vi "SR Speckle.vi"() -> ()   [LabVIEW 2012]
uses:
  user.lib/SpectralRadar.llb/Coloring.lvclass
  user.lib/SpectralRadar.llb/Colored Data.lvclass
  user.lib/SpectralRadar.llb/Colorscheme Selection.ctl
  user.lib/SpectralRadar.llb/Data.lvclass
  user.lib/SpectralRadar.llb/Specle Variance Type.ctl
  <vilib>/Utility/error.llb/DialogType.ctl
  user.lib/SpectralRadar.llb/Coloring Byteorder.ctl
  user.lib/SpectralRadar.llb/Probe Parameter Int Selection.ctl
  user.lib/SpectralRadar.llb/Processing Parameter Int Selection.ctl
  user.lib/SpectralRadar.llb/Data Export Format Selection.ctl
  user.lib/SpectralRadar.llb/Colored Data Export Format Selection.ctl
  user.lib/SpectralRadar.llb/Normal Direction Selection.ctl
  user.lib/SpectralRadar.llb/Calibration Selection.ctl
  user.lib/SpectralRadar.llb/Data Analyzation Selection.ctl
  user.lib/SpectralRadar.llb/set Complex Scan Output.vi
  user.lib/SpectralRadar.llb/set Scan Output.vi
  user.lib/SpectralRadar.llb/display Data 2D.vi
  user.lib/SpectralRadar.llb/OCT Device.lvclass
  user.lib/SpectralRadar.llb/LabVIEW Helper.lvlib
  user.lib/SpectralRadar.llb/Processing.lvclass
  user.lib/SpectralRadar.llb/Probe.lvclass
  user.lib/SpectralRadar.llb/Scan Pattern.lvclass
  user.lib/SpectralRadar.llb/Settings.lvclass
  user.lib/SpectralRadar.llb/Raw Data.lvclass
  user.lib/SpectralRadar.llb/FileSelection.lvlib
  user.lib/SpectralRadar.llb/Complex Data.lvclass
  user.lib/SpectralRadar.llb/Speckle Variance.lvclass
  user.lib/SpectralRadar.llb/Post Processing.lvlib
  user.lib/SpectralRadar.llb/FullRange.lvclass
panel:
  in  "Filter 3":bool
  in  "Filter 2":bool
  in  "Filter":bool
  in  "Filter Options":bool
  in  "Variance Type":T1
  in  "Averaging Axially":i32=1 min=1 max=10 step=1
  in  "Averaging Fast Axis":i32=1 min=1 max=10 step=1
  in  "Averaging Slow Axis":i32=3 min=1 max=10 step=1
  out "Volume Variance":refnum<class "Data.lvclass">
  out "Volume Mean":refnum<class "Data.lvclass">
  in  "Opacity":sgl(slide) scale=0.0..1.0
  in  "Shift Y [mm]":dbl
  in  "Shift X [mm]":dbl
  in  "Color Scheme":T2
  in  "Options":bool
  out "Colored Data":refnum<class "Colored Data.lvclass">
  out "Coloring":refnum<class "Coloring.lvclass">
  in  "Angle [rad]":dbl
  in  "Averaging-Binning-Ratio":dbl(slide) caption="Averaging vs. Binning" min=0.0 max=1.0 step=1.0
  in  "Averaging*Binning":i32(slide)=1 caption="Quality" min=1 max=200 step=1 scale=1.0..200.0
  out "AutoSafe":bool
  out "Progress":i32(slide) max=20 scale=0.0..384.0
  in  "Tab Control":enum32{"B-Scan"}(tab)
  out "Variance Frame":sgl[][](graph)
  in  "Variance Boundaries":cluster{sgl, sgl}(slide)={72.22738, 40.64965} scale=0.0..144.0705108642578
  in  "Boundries":cluster{sgl, sgl}(slide)={72.22738, 40.64965} scale=-20.0..150.0
  out "Mean Frame":sgl[][](graph)
  in  "X":dbl(slide) max=2.0 scale=0.0..2.0
  in  "Y":dbl(slide) max=3.0 scale=0.0..2.0
  in  "Z":dbl(slide) max=1.600000023841858 scale=0.0..5.12 scale format="%#_2g"
  in  "Export Format":T3(ring)
  out "Image":T4(plugin-control)
  out "Reference Intensity":sgl(slide) min=0 max=1 scale=0.0..1.0
  in  "Brightness":sgl(slide)=0.49673203 caption="Sharpness" min=0 max=1 scale=0.0..1.0
  in  "Contrast":sgl(slide)=0.53594774 caption="Sharpness" min=0 max=1 scale=0.0..1.0
  in  "Saturation":sgl(slide)=0.5294118 caption="Sharpness" min=0 max=1 scale=0.0..1.0
  in  "Light":i32(slide) min=0 max=100 step=1 scale=0.0..100.0
  in  "Description":string
  in  "Test Mode":bool
  out "Test Mode Indicator":bool
  in  "Window":T5(ring)
  out "FrameRate":sgl format="%#_3g"
  out "SpacingZ":dbl
  in  "Range Y [mm]":dbl=3.5999999046325684 caption="Bereich [mm]" min=0.0 max=10.0 step=0.05000000074505806 format="%_3f"
  out "Spacing Y [µm]":dbl=40.0 min=1.0 max=500.0 step=1.0 format="%#_3g"
  in  "Number Scans Y":i32=50 min=10 max=1000 step=1
  in  "Save":bool
  in  "Recalibrate":bool
  in  "Range X [mm]":dbl=2.5999999046325684 caption="Bereich [mm]" min=0.05000000074505806 max=10.0 step=0.05000000074505806 format="%_3f"
  out "Spacing X [µm]":dbl=2.0 min=1.0 max=500.0 step=1.0 format="%#_3g"
  in  "Number Scans X":i32=500 min=100 max=2000 step=1
  in  "Measure":bool
  in  "QuitApp":bool
  # "Stability"
  # "SNR"
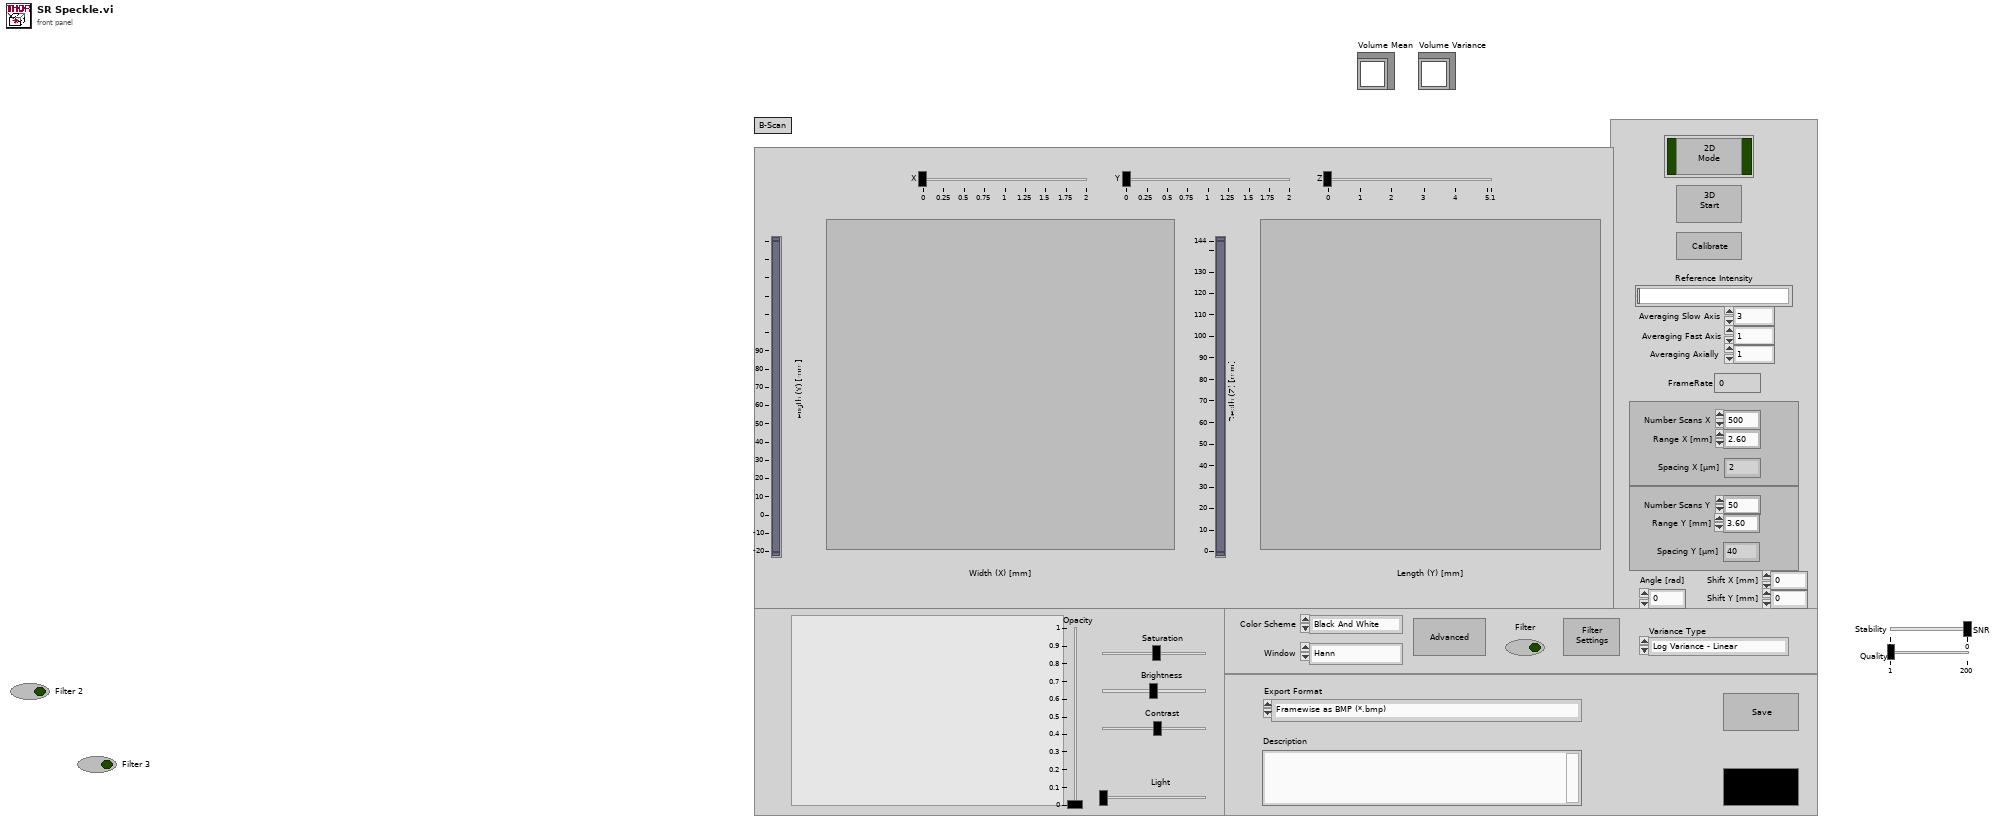
[diagram p1: front panel]
types:
  T1 = typedef "Speckle Variance.lvclass/Specle Variance Type.ctl" = enum16{"Log Variance - Linear", "Log Variance - Log", "Linear Variance - Linear", "Linear Variance - Log", "Complex Variance - Linear", "Complex Variance - Log"}
  T2 = typedef "Coloring.lvclass/Colorscheme Selection.ctl" = enum16{"Black And White", "Inverted Black And White", "Color", "Black and Orange", "Black and Red", "Doppler Phase Coloring"}
  T3 = enum16{"Framewise as BMP (*.bmp)", "Framewise as JPG (*.jpg)", "Framewise as PNG (*.png)", "Raw binary floating point (*.raw)", "VFF (*.vff)", "VTK (*.vtk)", "Flexible Image Transport System (*.fits)"}
  T4 = typedef "IMAQ Image.ctl" = refnum<image>
  T5 = enum16{"Hann", "Hamming", "Gauss", "Tapered Cosine", "Blackman", "4 Term B-Harris"}
  T6 = typedef "Coloring.lvclass/Coloring Byteorder.ctl" = enum16{"RGBA32", "BGRA32", "ARGB32", ""}
  T7 = enum16{"Full Well Capacity", "z Spacing", "z Range", "Dynamc Range Min [dB]", "Dynamic Range Low [dB]", "Dynamic Range High [dB]", "Dynamic Range Max [dB]"}
  T8 = typedef "Processing.lvclass/Processing Parameter Int Selection.ctl" = enum32{"Spectrum Averaging", "A-Scan Averaging", "B-Scan Averaging", "Zero Padding", "Number of Threads", "Fourier Averaging"}
  T9 = typedef "Probe.lvclass/Probe Parameter Int Selection.ctl" = enum16{"Apodization Cycles", "Oversampling", "Oversampling Slow Axis", "Speckle Reduction"}
  T10 = typedef "Data.lvclass/Data Export Format Selection.ctl" = enum16{"SRM (Spectral Radar Metafile)", "RAW", "CSV", "TXT", "Table TXT", "Fits", "VFF", "VTK", "TIFF"}
  T11 = typedef "Colored Data.lvclass/Colored Data Export Format Selection.ctl" = enum16{"SRM (Spectral Radar Metafile)", "RAW", "BMP", "PNG", "JPG", "PDF", "TIFF"}
  T12 = enum16{"Asynchronous Continuous", "Asynchronous Finite", "Synchronous"}
  T13 = typedef "Data.lvclass/Normal Direction Selection.ctl" = enum16{"Direction 1", "Direction 2", "Direction 3"}
  T14 = enum8{"Enabled", "Disabled", "Disabled and Grayed Out"}
  T15 = typedef "Processing.lvclass/Calibration Selection.ctl" = enum16{"Offset Errors", "Apodization Spectrum", "Apodization Vector", "Dispersion", "Chirp", "Extended Adjust", "Fixed Pattern"}
  T16 = typedef "Data.lvclass/Data Analyzation Selection.ctl" = enum16{"Min", "Mean", "Max"}
  T17 = typedef "DialogType.ctl" = u16
  T18 = typedef "Image Type" = u32
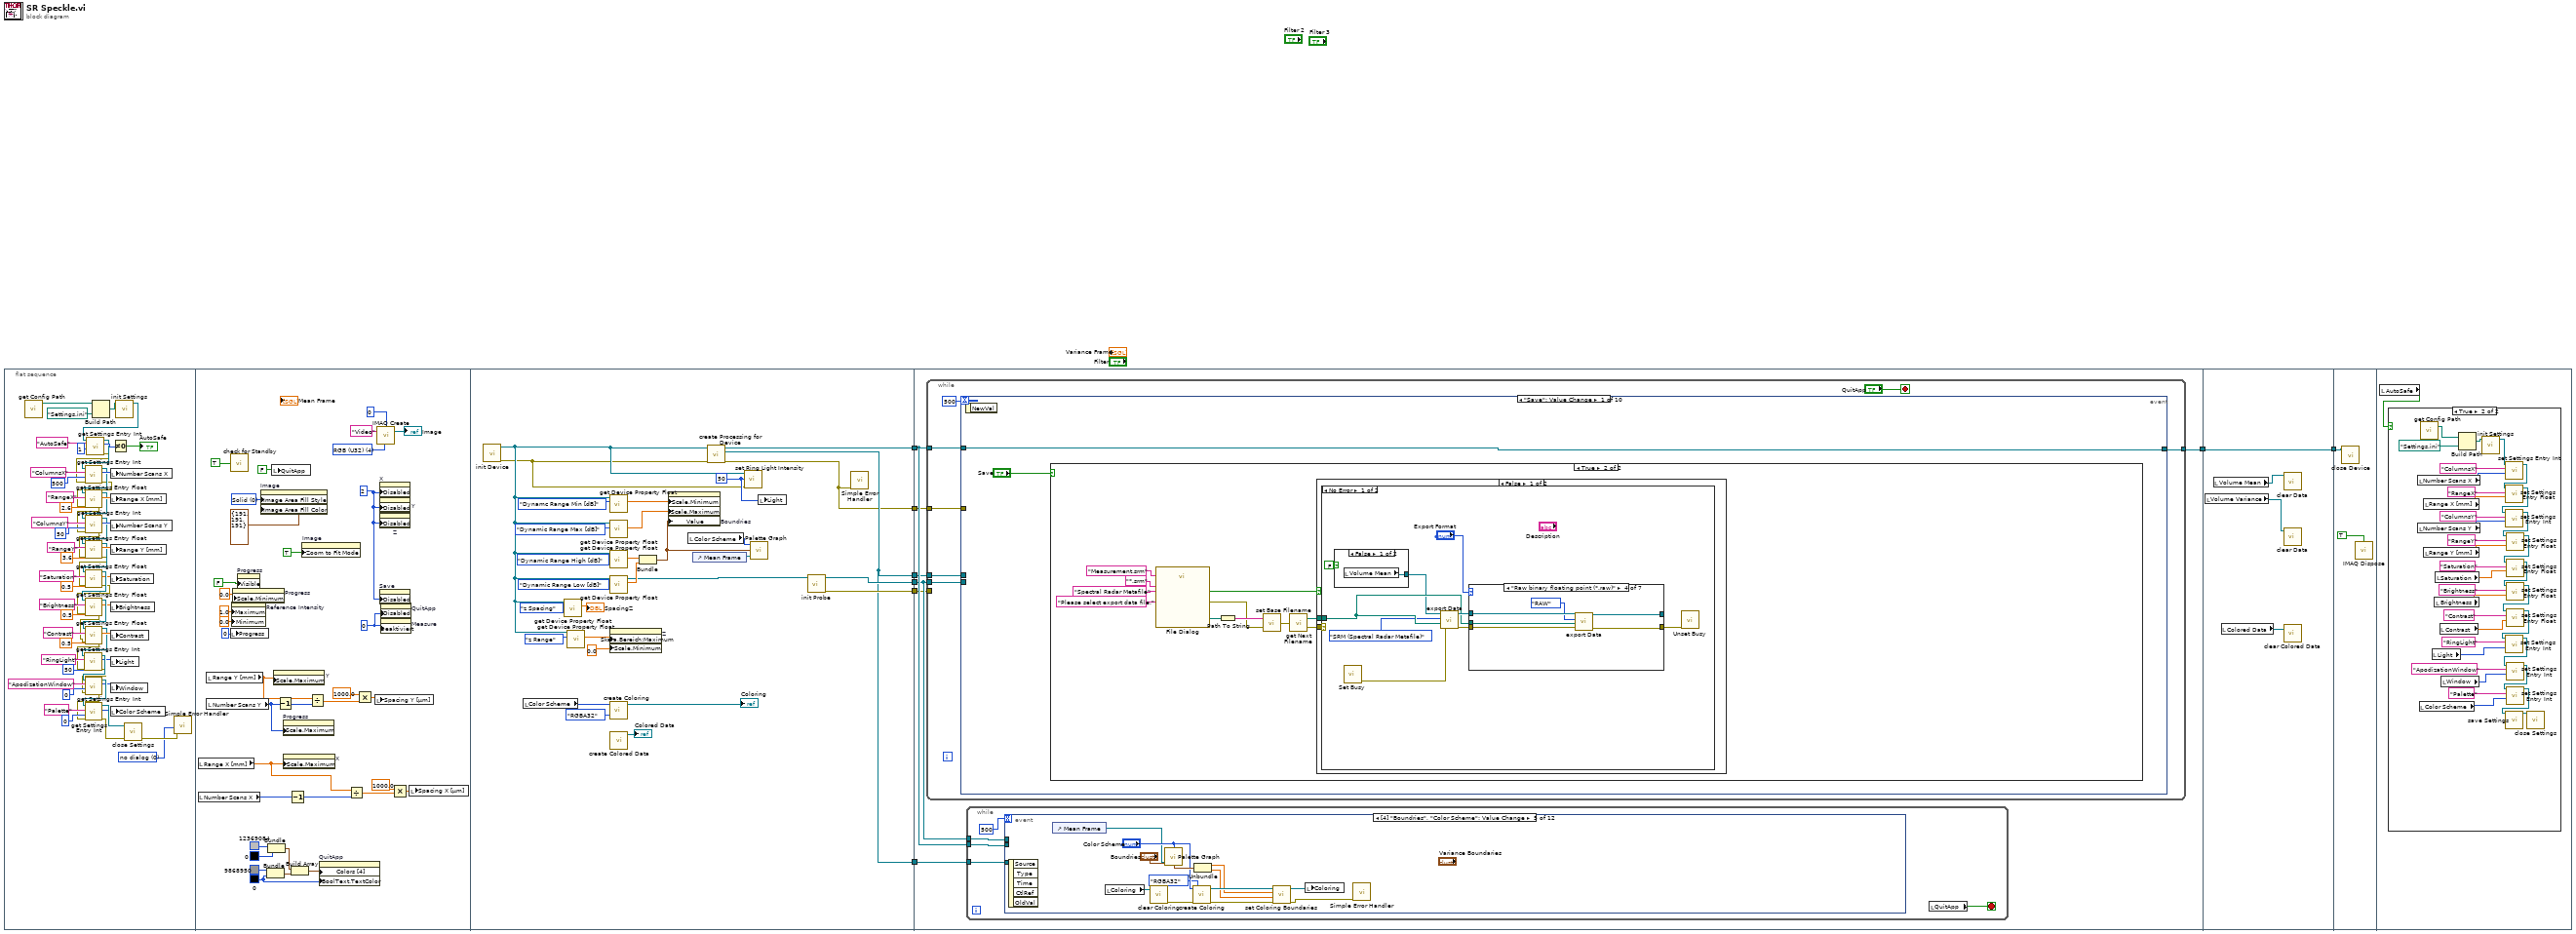
[diagram p0: block diagram]
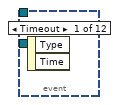
[diagram p2: hidden frame]
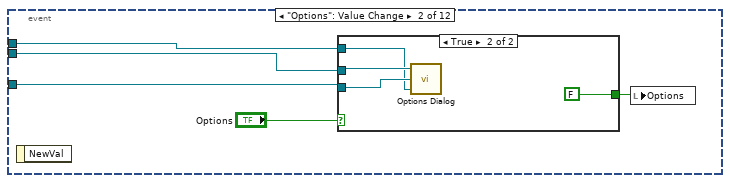
[diagram p3: hidden frame]
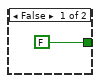
[diagram p4: hidden frame]
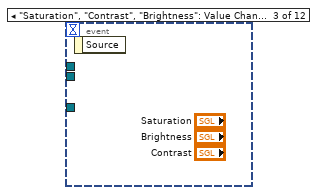
[diagram p5: hidden frame]
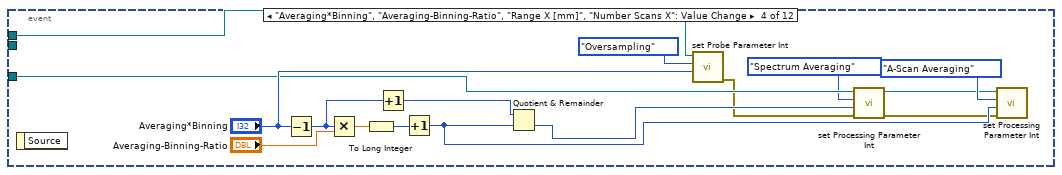
[diagram p6: hidden frame]
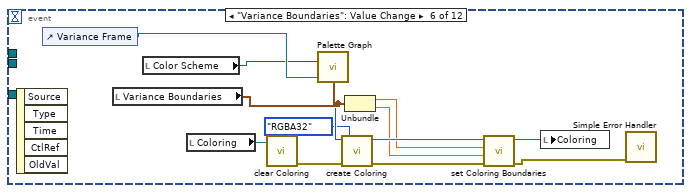
[diagram p7: hidden frame]
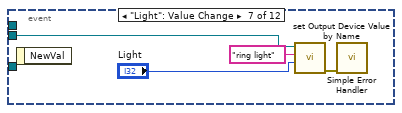
[diagram p8: hidden frame]
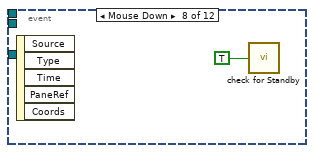
[diagram p9: hidden frame]
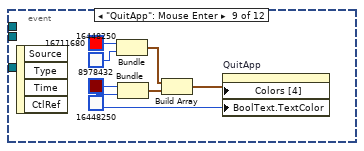
[diagram p10: hidden frame]
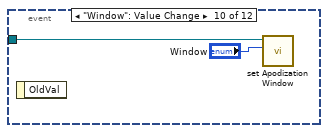
[diagram p11: hidden frame]
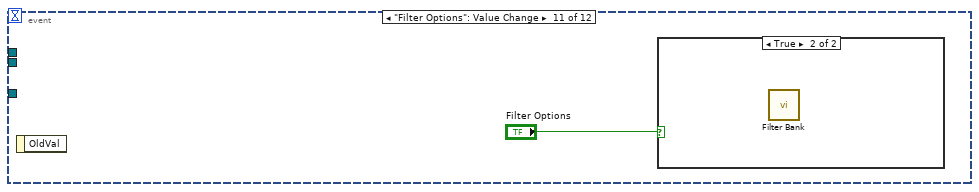
[diagram p12: hidden frame]
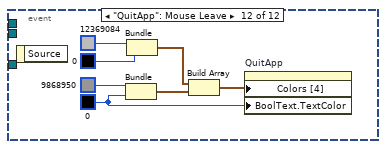
[diagram p14: hidden frame]
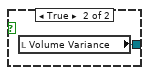
[diagram p16: hidden frame]
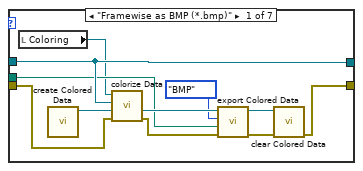
[diagram p17: hidden frame]
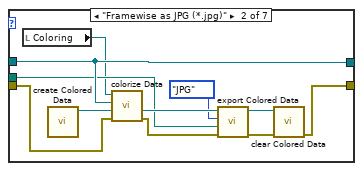
[diagram p18: hidden frame]
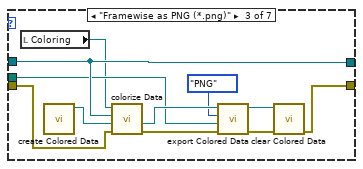
[diagram p19: hidden frame]
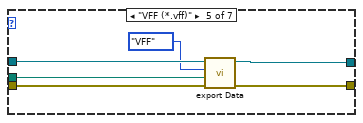
[diagram p20: hidden frame]
diagram:
  n1 = flat-sequence {
    tunnel: [w117] -> w8
    tunnel: [w118] -> w5
    tunnel: [w131] -> w4
    tunnel: [w118] -> w3
    tunnel: [w116] -> w2
    tunnel: [w129] -> w1
    tunnel: w8 -> [w140]
    tunnel: [w141] -> w6
    tunnel: w5 -> [w139]
    tunnel: w4 -> [w137]
    tunnel: w3 -> [w138]
    tunnel: w2 -> [w136]
    tunnel: w1 -> [w135]
    tunnel: [w747] -> w7
    tunnel: w6 -> [w747]
    tunnel: w7 -> [w749]
    frame #0 {
      w10 = T17 0 items=["no dialog", "OK message", "continue or stop message", "OK message + warnings", "continue/stop + warnings"] ("type of dialog (OK msg:1)")
      n2 = call "get Config Path.vi"() -> ("Path"=w20:path)  [unwired: 1 in, 1 out]
      n3 = Build Path(base path=w20, name or relative path=path "Settings.ini" ("Relative \"SpectralRadar.ini\" Path")) -> (appended path=w61:path)
      n4 = call "init Settings.vi"("Path to settings file"=w61) -> ("Settings"=w30:refnum<class "Settings.lvclass">)  [unwired: 5 in, 1 out]
      n5 = call "get Settings Entry Int.vi"("Default Value"=1, "Node Name"="AutoSafe", "Settings"=w30) -> ("error out"=w23:errorcluster, "Value"=w33:i32, "Settings"=w29:refnum<class "Settings.lvclass">)  [unwired: 2 in]
      n6 = call "get Settings Entry Int.vi"("error in (no error)"=w23, "Default Value"=500, "Node Name"="ColumnsX", "Settings"=w29) -> ("error out"=w22:errorcluster, "Value"=w60:i32, "Settings"=w46:refnum<class "Settings.lvclass">)  [unwired: 1 in]
      n7 = call "get Settings Entry Float.vi"("error in (no error)"=w22, "Default Value"=2.6, "Node Name"="RangeX", "Settings"=w46) -> ("error out"=w21:errorcluster, "Value"=w59:dbl, "Settings"=w45:refnum<class "Settings.lvclass">)  [unwired: 1 in]
      n8 = call "get Settings Entry Int.vi"("error in (no error)"=w21, "Default Value"=50, "Node Name"="ColumnsY", "Settings"=w45) -> ("error out"=w19:errorcluster, "Value"=w58:i32, "Settings"=w44:refnum<class "Settings.lvclass">)  [unwired: 1 in]
      n9 = call "get Settings Entry Float.vi"("error in (no error)"=w19, "Default Value"=3.6, "Node Name"="RangeY", "Settings"=w44) -> ("error out"=w18:errorcluster, "Value"=w57:dbl, "Settings"=w43:refnum<class "Settings.lvclass">)  [unwired: 1 in]
      n10 = call "get Settings Entry Float.vi"("error in (no error)"=w18, "Default Value"=0.5, "Node Name"="Saturation", "Settings"=w43) -> ("error out"=w17:errorcluster, "Value"=w36:dbl, "Settings"=w42:refnum<class "Settings.lvclass">)  [unwired: 1 in]
      n11 = call "get Settings Entry Float.vi"("error in (no error)"=w17, "Default Value"=0.5, "Node Name"="Brightness", "Settings"=w42) -> ("error out"=w16:errorcluster, "Value"=w37:dbl, "Settings"=w41:refnum<class "Settings.lvclass">)  [unwired: 1 in]
      n12 = call "get Settings Entry Float.vi"("error in (no error)"=w16, "Default Value"=0.5, "Node Name"="Contrast", "Settings"=w41) -> ("error out"=w15:errorcluster, "Value"=w38:dbl, "Settings"=w28:refnum<class "Settings.lvclass">)  [unwired: 1 in]
      n13 = call "get Settings Entry Int.vi"("error in (no error)"=w15, "Default Value"=50, "Node Name"="RingLight", "Settings"=w28) -> ("error out"=w14:errorcluster, "Value"=w24:i32, "Settings"=w26:refnum<class "Settings.lvclass">)  [unwired: 1 in]
      n14 = call "get Settings Entry Int.vi"("error in (no error)"=w14, "Default Value"=0, "Node Name"="ApodizationWindow", "Settings"=w26) -> ("error out"=w13:errorcluster, "Value"=w39:i32, "Settings"=w40:refnum<class "Settings.lvclass">)  [unwired: 1 in]
      n15 = call "get Settings Entry Int.vi"("error in (no error)"=w13, "Default Value"=0, "Node Name"="Palette", "Settings"=w40) -> ("error out"=w12:errorcluster, "Value"=w9:i32, "Settings"=w35:refnum<class "Settings.lvclass">)  [unwired: 1 in]
      n16 = local write "Number Scans X"(w60) -> ()
      n17 = local write "Range X [mm]"(w59) -> ()
      n18 = local write "Number Scans Y"(w58) -> ()
      n19 = local write "Range Y [mm]"(w57) -> ()
      n20 = local write "Saturation"(w36) -> ()
      n21 = local write "Brightness"(w37) -> ()
      n22 = local write "Contrast"(w38) -> ()
      n23 = local write "Light"(w24) -> ()
      n24 = local write "Window"(w39) -> ()
      n25 = local write "Color Scheme"(w9) -> ()
      n26 = Not Equal To 0?(x=w33) -> (x != 0?=→"AutoSafe":bool)
      n27 = call "close Settings.vi"("error in (no error)"=w12, "Settings"=w35) -> ("error out"=w11:errorcluster)  [unwired: 5 in]
      n28 = call <vilib>:"Simple Error Handler.vi"("type of dialog (OK msg:1)"=w10, "error in (no error)"=w11) -> ()  [unwired: 3 in, 5 out]
    }
    frame #1 {
      w72 = T18 4 items=["Grayscale (U8)", "Grayscale (I16)", "Grayscale (SGL)", "Complex (CSG)", "RGB (U32)", "HSL (U32)", "RGB (U64)", "Grayscale (U16)"] ("Image Type")
      w76 = u8 0 ("Deaktiviert")
      w89 = u8 2 ("Disabled")
      w97 = u32 0
      w102 = u32 0 items=["Default"=3, "Solid"=0, "Hatch"=2] ("Image Area:Background:Fill Style")
      n29 = local read "Range X [mm]"() -> (w77:dbl)
      n30 = local read "Number Scans X"() -> (w79:i32)
      n31 = local read "Range Y [mm]"() -> (w84:dbl)
      n32 = local read "Number Scans Y"() -> (w85:i32)
      n33 = call "check for Standby.vi"("ResetTimer"=TRUE) -> ()  [unwired: 2 out]
      n34 = local write "Progress"(0 ("Progress")) -> ()
      n35 = property on="Reference Intensity" class="Slide (strict)"("Maximum"=1.0 ("Data Entry Limits:Maximum"), "Minimum"=0.0 ("Data Entry Limits:Minimum")) -> ()  [unwired: 2 in, 2 out]
      n36 = property on="Progress" class="Slide (strict)"("Scale.Minimum"=0.0 ("Skalieren.Bereich:Minimum")) -> ()  [unwired: 2 in, 2 out]
      n37 = property on="Progress" class="Slide (strict)"("Visible"=FALSE ("Sichtbar")) -> ()  [unwired: 2 in, 2 out]
      n38 = property on="Image" class="ImageControl"("Image Area Fill Style"=w102, "Image Area Fill Color"=cluster{"Red":u8, "Green":u8, "Blue":u8} {"Red"=191, "Green"=191, "Blue"=191} ("Image Area:Background:Fill Color")) -> ()  [unwired: 2 in, 2 out]
      n39 = Bundle(u32 9868950, w97) -> (w95:cluster{u32, u32})  [unwired: 1 in]
      n40 = Bundle(u32 12369084, u32 0) -> (w94:cluster{u32, u32})  [unwired: 1 in]
      n41 = local write "QuitApp"(FALSE ("QuitApp")) -> ()
      n42 = property on="Y" class="Slide (strict)"("Scale.Maximum"=w84) -> ()  [unwired: 2 in, 2 out]
      n43 = Decrement(x=w85) -> (x-1=w83:i32)
      n44 = property on="Progress" class="Slide (strict)"("Scale.Maximum"=w85) -> ()  [unwired: 2 in, 2 out]
      n45 = property on="X" class="Slide (strict)"("Scale.Maximum"=w77) -> ()  [unwired: 2 in, 2 out]
      n46 = Decrement(x=w79) -> (x-1=w78:i32)
      n47 = Build Array(w94, w95) -> (w96:cluster{u32, u32}[])
      n48 = property on="Image" class="ImageControl"("Zoom to Fit Mode"=TRUE) -> ()  [unwired: 2 in, 2 out]
      n49 = Divide(x=w84, y=w83) -> (x/y=w87:dbl)
      n50 = property on="QuitApp" class="Bool (strict)"("Colors [4]"=w96, "BoolText.TextColor"=w97) -> ()  [unwired: 2 in, 2 out]
      n51 = Divide(x=w77, y=w78) -> (x/y=w81:dbl)
      n52 = Multiply(x=1000.0, y=w87) -> (x*y=w88:dbl)
      n53 = local write "Spacing Y [µm]"(w88) -> ()
      n54 = call "IMAQ Create"("Border Size"=0, "Image Name"="Video", "Image Type"=w72) -> ("New Image"=→"Image":T4)  [unwired: 2 in, 1 out]
      n55 = property on="X" class="Slide (strict)"("Disabled"=w89) -> ()  [unwired: 2 in, 2 out]
      n56 = property on="Y" class="Slide (strict)"("Disabled"=w89) -> ()  [unwired: 2 in, 2 out]
      n57 = property on="Z" class="Slide (strict)"("Disabled"=w89) -> ()  [unwired: 2 in, 2 out]
      n58 = property on="Save" class="Bool"("Disabled"=w89) -> ()  [unwired: 2 in, 2 out]
      n59 = property on="QuitApp" class="Bool (strict)"("Disabled"=w76) -> ()  [unwired: 2 in, 2 out]
      n60 = property on="Measure" class="Bool"("Deaktiviert"=w76) -> ()  [unwired: 2 in, 2 out]
      n61 = Multiply(x=sgl 1000.0, y=w81) -> (x*y=w82:dbl)
      n62 = local write "Spacing X [µm]"(w82) -> ()
    }
    frame #2 {
      w134 = 50 ("Intensity[%]")
      n63 = call "init Device.vi"() -> ("error out"=w106:errorcluster, "OCTDevice"=w110:refnum<class "OCT Device.lvclass">)  [unwired: 6 in]
      n64 = local read "Color Scheme"() -> (w108:T2)
      n65 = call "get Device Property Float.vi"("Device Property Float Selection"=T7."z Spacing", "OCTDevice"=w110) -> ("Value"=→"SpacingZ":dbl)  [unwired: 3 in, 2 out]
      n66 = call "get Device Property Float.vi"("Device Property Float Selection"=T7."z Range", "OCTDevice"=w110) -> ("Value"=w114:dbl)  [unwired: 3 in, 2 out]
      n67 = call "get Device Property Float.vi"("Device Property Float Selection"=T7."Dynamc Range Min [dB]", "OCTDevice"=w110) -> ("Value"=w125:dbl)  [unwired: 3 in, 2 out]
      n68 = call "get Device Property Float.vi"("Device Property Float Selection"=T7."Dynamic Range Max [dB]", "OCTDevice"=w110) -> ("Value"=w124:dbl)  [unwired: 3 in, 2 out]
      n69 = call "get Device Property Float.vi"("Device Property Float Selection"=T7."Dynamic Range High [dB]", "OCTDevice"=w110) -> ("Value"=w120:dbl)  [unwired: 3 in, 2 out]
      n70 = call "get Device Property Float.vi"("Device Property Float Selection"=T7."Dynamic Range Low [dB]", "OCTDevice"=w110) -> ("Value"=w119:dbl, "OCTDevice"=w111:refnum<class "OCT Device.lvclass">)  [unwired: 3 in, 1 out]
      n71 = call "create Coloring.vi"("Color Byte Order"=Coloring_Byteorder."RGBA32", "Color Table Selection"=w108) -> ("Coloring"=→"Coloring":refnum<class "Coloring.lvclass">)  [unwired: 4 in, 1 out]
      n72 = property on="Z" class="Slide (strict)"("Skala.Bereich:Maximum"=w114, "Scale.Minimum"=0.0 ("Scale.Range:Minimum")) -> ()  [unwired: 2 in, 2 out]
      n73 = call "create Colored Data.vi"() -> ("Colored Data"=→"Colored Data":refnum<class "Colored Data.lvclass">)  [unwired: 6 in, 1 out]
      n74 = Bundle("Value"=w120, "Value"=w119) -> (w132:cluster{"Value":dbl, "Value":dbl})  [unwired: 1 in]
      n75 = property on="Boundries" class="Slide (strict)"("Scale.Minimum"=w125, "Scale.Maximum"=w124, "Value"=w132) -> ()  [unwired: 2 in, 2 out]
      n76 = local read "Color Scheme"() -> (w109:T2)
      n77 = control-ref of="Mean Frame"() -> (w133:refnum<vi>)
      n78 = call "create Processing for Device.vi"("error in (no error)"=w106, "OCTDevice"=w110) -> ("error out"=w116:errorcluster, "Processing"=w118:refnum<class "Processing.lvclass">, "OCTDevice"=w117:refnum<class "OCT Device.lvclass">)  [unwired: 3 in]
      n79 = call "set Ring Light Intensity.vi"("error in (no error)"=w106, "Intensity[%]"=w134, "OCTDevice"=w110) -> ()  [unwired: 3 in, 2 out]
      n80 = call "Palette Graph.vi"("Reference to the B-scan Graph"=w133, "Boundaries"=w132, "Color Scheme"=w109) -> ()
      n81 = local write "Light"(w134) -> ()
      n82 = call "init Probe.vi"("OCT Device"=w111) -> ("error out"=w129:errorcluster, "GalvoControl"=w131:refnum<class "Probe.lvclass">)  [unwired: 5 in]
      n83 = call <vilib>:"Simple Error Handler.vi"("error in (no error)"=w116) -> ()  [unwired: 4 in, 5 out]
    }
    frame #3 {
      n84 = while {
        tunnel: w140 -> [w222]
        tunnel: [w223] -> w141
        tunnel: w139 -> [w221]
        tunnel: w137 -> [w220]
        tunnel: w136 -> [w219]
        tunnel: w135 -> [_]
        stop <- "QuitApp" stop-if-true
        n85 = event shown="[0] \"Save\": Value Change" {
          selector: _ -> [_ _ _ _ _ _ _ _ _ _]
          dyn-events: _ -> [_ _ _ _ _ _ _ _ _ _]
          timeout: 500 -> [_ _ _ _ _ _ _ _ _ _]
          tunnel: w222 -> [w227 w316 w324 w488 w598 w606 w612 w651 w695 w737]
          tunnel: [w227 w314 w323 w486 w598 w606 w612 w651 w695 w737] -> w223
          tunnel: w221 -> [_ _ w320 w484 _ _ w611 _ _ _]
          tunnel: w220 -> [_ _ w322 w485 _ _ _ _ _ _]
          tunnel: w219 -> [_ _ w319 _ _ _ _ _ _ _]
          event "Save": Value Change {
            n86 = event-data() -> ()  [unwired: 1 in, 1 out]
            n87 = case shown="True" "Save" {
              frame False {
              }
              frame True {
                n88 = call "File Dialog"("prompt"="Please select export data file.", "default name"="Measurement.srm", "pattern (all files)"="*.srm", "pattern label"="Spectral Radar Metafile") -> ("selected path"=w232:path, "cancelled"=w230:bool, "error out"=w229:errorcluster)  [unwired: 8 in, 1 out]
                n89 = Path To String(path=w232) -> (string=w231:string)
                n90 = call "set Base Filename.vi"("error in (no error)"=w229, "Base"=w231) -> ("error out"=w238:errorcluster)
                n91 = call "get Next Filename.vi"("error in (no error)"=w238) -> ("Next File Name"=w237:path, "error out"=w228:errorcluster)
                n92 = case shown="False" w230 {
                  tunnel: w237 -> [w240 _]
                  tunnel: w228 -> [w239 _]
                  frame False {
                    n93 = case shown="No Error" w239 {
                      tunnel: w240 -> [w244 _]
                      frame No Error {
                        n94 = case shown="False" FALSE {
                          tunnel: [w250 w251] -> w242
                          frame False {
                            n95 = local read "Volume Mean"() -> (w250:refnum<class "Data.lvclass">)
                          }
                          frame True {
                            n96 = local read "Volume Variance"() -> (w251:refnum<class "Data.lvclass">)
                          }
                        }
                        n97 = call <vilib>:"Set Busy.vi"() -> ("error out"=w246:errorcluster)  [unwired: 10 in, 1 out]
                        n98 = call "export Data.vi"("error in (no error)"=w246, "Export File"=w244, "Data Export Format Selection"=Data_Export_Format_Selection."SRM (Spectral Radar Metafile)" ("Data 2D Export Format Selection"), "Data in"=w242) -> ("error out"=w247:errorcluster, "Data out"=w248:refnum<class "Data.lvclass">)  [unwired: 2 in]
                        n99 = case shown="\"Raw binary floating point (*.raw)\"" "Export Format" {
                          tunnel: w248 -> [w262 w273 w284 w290 w296 w301 w308]
                          tunnel: [w262 w273 w284 w289 w295 w302 w307] -> _
                          tunnel: w244 -> [w259 w270 w281 w285 w292 w298 w304]
                          tunnel: w247 -> [w256 w267 w278 w288 w294 w300 w306]
                          tunnel: [w253 w264 w275 w287 w293 w299 w305] -> w245
                          frame "Framewise as BMP (*.bmp)" {
                            n100 = local read "Coloring"() -> (w252:refnum<class "Coloring.lvclass">)
                            n101 = call "create Colored Data.vi"() -> ("Colored Data"=w261:refnum<class "Colored Data.lvclass">)  [unwired: 6 in, 1 out]
                            n102 = call "colorize Data.vi"("error in (no error)"=w256, "Colored Data"=w261, "Data"=w262, "Coloring in"=w252) -> ("error out"=w255:errorcluster, "Colored Data"=w260:refnum<class "Colored Data.lvclass">)  [unwired: 2 out]
                            n103 = call "export Colored Data.vi"("error in (no error)"=w255, "File Name"=w259, "Colored Data Export Format Selection"=Colored_Data_Export_Format_Selection."BMP", "Colored Data in"=w260) -> ("error out"=w254:errorcluster, "Colored Data out"=w257:refnum<class "Colored Data.lvclass">)  [unwired: 2 in]
                            n104 = call "clear Colored Data.vi"("error in (no error)"=w254, "Colored Data"=w257) -> ("error out"=w253:errorcluster)  [unwired: 5 in]
                          }
                          frame "Framewise as JPG (*.jpg)" {
                            n105 = local read "Coloring"() -> (w263:refnum<class "Coloring.lvclass">)
                            n106 = call "create Colored Data.vi"() -> ("Colored Data"=w272:refnum<class "Colored Data.lvclass">)  [unwired: 6 in, 1 out]
                            n107 = call "colorize Data.vi"("error in (no error)"=w267, "Colored Data"=w272, "Data"=w273, "Coloring in"=w263) -> ("error out"=w266:errorcluster, "Colored Data"=w271:refnum<class "Colored Data.lvclass">)  [unwired: 2 out]
                            n108 = call "export Colored Data.vi"("error in (no error)"=w266, "File Name"=w270, "Colored Data Export Format Selection"=Colored_Data_Export_Format_Selection."JPG", "Colored Data in"=w271) -> ("error out"=w265:errorcluster, "Colored Data out"=w268:refnum<class "Colored Data.lvclass">)  [unwired: 2 in]
                            n109 = call "clear Colored Data.vi"("error in (no error)"=w265, "Colored Data"=w268) -> ("error out"=w264:errorcluster)  [unwired: 5 in]
                          }
                          frame "Framewise as PNG (*.png)" {
                            n110 = local read "Coloring"() -> (w274:refnum<class "Coloring.lvclass">)
                            n111 = call "create Colored Data.vi"() -> ("Colored Data"=w283:refnum<class "Colored Data.lvclass">)  [unwired: 6 in, 1 out]
                            n112 = call "colorize Data.vi"("error in (no error)"=w278, "Colored Data"=w283, "Data"=w284, "Coloring in"=w274) -> ("error out"=w277:errorcluster, "Colored Data"=w282:refnum<class "Colored Data.lvclass">)  [unwired: 2 out]
                            n113 = call "export Colored Data.vi"("error in (no error)"=w277, "File Name"=w281, "Colored Data Export Format Selection"=Colored_Data_Export_Format_Selection."PNG", "Colored Data in"=w282) -> ("error out"=w276:errorcluster, "Colored Data out"=w279:refnum<class "Colored Data.lvclass">)  [unwired: 2 in]
                            n114 = call "clear Colored Data.vi"("error in (no error)"=w276, "Colored Data"=w279) -> ("error out"=w275:errorcluster)  [unwired: 5 in]
                          }
                          frame "Raw binary floating point (*.raw)" {
                            n115 = call "export Data.vi"("error in (no error)"=w288, "Export File"=w285, "Data Export Format Selection"=Data_Export_Format_Selection."RAW" ("Data 2D Export Format Selection"), "Data in"=w290) -> ("error out"=w287:errorcluster, "Data out"=w289:refnum<class "Data.lvclass">)  [unwired: 2 in]
                          }
                          frame "VFF (*.vff)" {
                            n116 = call "export Data.vi"("error in (no error)"=w294, "Export File"=w292, "Data Export Format Selection"=Data_Export_Format_Selection."VFF" ("Data 2D Export Format Selection"), "Data in"=w296) -> ("error out"=w293:errorcluster, "Data out"=w295:refnum<class "Data.lvclass">)  [unwired: 2 in]
                          }
                          frame "VTK (*.vtk)" {
                            n117 = call "export Data.vi"("error in (no error)"=w300, "Export File"=w298, "Data Export Format Selection"=Data_Export_Format_Selection."VTK" ("Data 2D Export Format Selection"), "Data in"=w301) -> ("error out"=w299:errorcluster, "Data out"=w302:refnum<class "Data.lvclass">)  [unwired: 2 in]
                          }
                          frame "Flexible Image Transport System (*.fits)" {
                            n118 = call "export Data.vi"("error in (no error)"=w306, "Export File"=w304, "Data Export Format Selection"=Data_Export_Format_Selection."Table TXT" ("Data 2D Export Format Selection"), "Data in"=w308) -> ("error out"=w305:errorcluster, "Data out"=w307:refnum<class "Data.lvclass">)  [unwired: 2 in]
                          }
                        }
                        n119 = call <vilib>:"Unset Busy.vi"("error in (no error)"=w245) -> ()  [unwired: 10 in, 1 out]
                      }
                      frame Error {
                      }
                    }
                  }
                  frame True {
                  }
                }
              }
            }
          }
          event Timeout {
            n120 = event-data() -> ()  [unwired: 1 in, 1 out]
            n121 = call "check for Standby.vi"() -> ("TimeOut"=w318:bool)  [unwired: 1 in, 1 out]
            n122 = call "activate Standby.vi"("StandBy"=w318, "OCTDevice"=w316) -> ("OCTDevice"=w315:refnum<class "OCT Device.lvclass">)  [unwired: 4 in, 1 out]
            n123 = local read "Colored Data"() -> (w317:refnum<class "Colored Data.lvclass">)
            n124 = call "get Camera Image.vi"("Colored Data in"=w317, "OCTDevice in"=w315) -> ("error out"=w311:errorcluster, "Colored Data out"=w312:refnum<class "Colored Data.lvclass">, "OCTDevice out"=w314:refnum<class "OCT Device.lvclass">)  [unwired: 5 in]
            n125 = local read "Image"() -> (w313:T4)
            n126 = call "update Colored Data IMAQ Image.vi"("error in (no error)"=w311, "Image in"=w313, "Colored Data"=w312) -> ("error out"=w309:errorcluster, "Image out"=w310:T4)  [unwired: 2 in, 1 out]
            n127 = local write "Image"(w310) -> ()
            n128 = call <vilib>:"Clear Errors.vi"("error in (no error)"=w309) -> ()  [unwired: 6 in, 1 out]
          }
          event "Measure": Value Change {
            n129 = event-data() -> ()  [unwired: 1 in, 1 out]
            n130 = case shown="True" "Measure" {
              tunnel: w324 -> [w325 w350]
              tunnel: [w325 w354] -> w323
              tunnel: w322 -> [_ w353]
              tunnel: w320 -> [_ w352]
              tunnel: w319 -> [_ w351]
              frame False {
              }
              frame True {
                n131 = flat-sequence {
                  tunnel: w351 -> [w361]
                  tunnel: w352 -> [w362]
                  tunnel: w353 -> [w358]
                  tunnel: w350 -> [w363]
                  tunnel: [w363] -> w349
                  tunnel: [w357] -> w348
                  tunnel: [w362] -> w347
                  tunnel: [w361] -> w346
                  tunnel: ["Number Scans Y"] -> w345
                  tunnel: [w404] -> w344
                  tunnel: [w385] -> w343
                  tunnel: [w396] -> w342
                  tunnel: [w379] -> w341
                  tunnel: [w395] -> w340
                  tunnel: [w375] -> w339
                  tunnel: w349 -> [w392]
                  tunnel: w348 -> [w400]
                  tunnel: w347 -> [w396]
                  tunnel: w346 -> [_]
                  tunnel: [errorcluster {"status"=FALSE, "code"=0, "source"=""} ("error out")] -> w330
                  tunnel: [w377] -> w328
                  tunnel: [w426] -> w338
                  tunnel: w345 -> [w426]
                  tunnel: [w425] -> w337
                  tunnel: [w424] -> w336
                  tunnel: w344 -> [w424]
                  tunnel: w343 -> [w422]
                  tunnel: w342 -> [w421]
                  tunnel: w341 -> [w423]
                  tunnel: w340 -> [w420]
                  tunnel: w339 -> [w419]
                  tunnel: [w418] -> w335
                  tunnel: [w417] -> w334
                  tunnel: [w416] -> w333
                  tunnel: w330 -> [w415]
                  tunnel: [w414] -> w329
                  tunnel: w328 -> [w412]
                  tunnel: [w411] -> w327
                  tunnel: w338 -> [w482]
                  tunnel: [0 ("Progress")] -> w332
                  tunnel: [FALSE ("Sichtbar")] -> w331
                  tunnel: w337 -> [w479]
                  tunnel: [w478] -> w354
                  tunnel: w336 -> [w477]
                  tunnel: w335 -> [w474]
                  tunnel: w334 -> [_]
                  tunnel: w333 -> [w466]
                  tunnel: w329 -> [w465]
                  tunnel: w327 -> [w464]
                  tunnel: [0.0] -> w326
                  frame #0 {
                    n132 = local read "Volume Variance"() -> (w360:refnum<class "Data.lvclass">)
                    n133 = local read "Volume Mean"() -> (w359:refnum<class "Data.lvclass">)
                    n134 = call <vilib>:"Set Busy.vi"() -> ()  [unwired: 10 in, 2 out]
                    n135 = call "clear Data.vi"("Data"=w359) -> ()  [unwired: 6 in, 1 out]
                    n136 = call "clear Data.vi"("Data"=w360) -> ()  [unwired: 6 in, 1 out]
                    n137 = call "set Probe Parameter Int.vi"("Value"="Averaging Slow Axis", "Probe Parameter Int"=Probe_Parameter_Int_Selection."Oversampling Slow Axis", "GalvoControl"=w358) -> ("GalvoControl"=w357:refnum<class "Probe.lvclass">)  [unwired: 3 in, 1 out]
                  }
                  frame #1 {
                    w405 = u8 2 ("Deaktiviert")
                    w403 = u8 2
                    # "Expected\nA-Scan\nSize"
                    # "Surface"
                    # "Volume"
                    # "BScan"
                    n138 = local read "Averaging Slow Axis"() -> (w369:i32)
                    n139 = local read "Number Scans Y"() -> (w368:i32)
                    n140 = local read "Range X [mm]"() -> (w409:dbl)
                    n141 = local read "Range Y [mm]"() -> (w410:dbl)
                    n142 = local read "Colored Data"() -> (w394:refnum<class "Colored Data.lvclass">)
                    n143 = local read "Range X [mm]"() -> (w402:dbl)
                    n144 = local read "Range Y [mm]"() -> (w401:dbl)
                    n145 = property on="Recalibrate" class="Bool"("Disabled"=w405) -> ()  [unwired: 2 in, 2 out]
                    n146 = property on="Save" class="Bool"("Disabled"=w405) -> ()  [unwired: 2 in, 2 out]
                    n147 = property on="QuitApp" class="Bool (strict)"("Disabled"=w405) -> ()  [unwired: 2 in, 2 out]
                    n148 = property on="Progress" class="Slide (strict)"("Visible"=TRUE ("Sichtbar")) -> ()  [unwired: 2 in, 2 out]
                    n149 = property on="Mean Frame" class="IntGraph (strict)"("XScale.NameLbl.Text"="Width (X) [mm]" ("X Scale.Name Label.Text"), "YScale.NameLbl.Text"="Depth (Z) [mm]" ("Y Scale.Name Label.Text")) -> ()  [unwired: 2 in, 2 out]
                    n150 = Multiply(x=w368, y=w369) -> (x*y=w367:i32)
                    n151 = call "get Camera Image.vi"("Colored Data in"=w394, "OCTDevice in"=w392) -> ("error out"=w380:errorcluster, "OCTDevice out"=w364:refnum<class "OCT Device.lvclass">)  [unwired: 5 in, 1 out]
                    n152 = property on="X" class="Slide (strict)"("Skala.Bereich:Maximum"=w409) -> ()  [unwired: 2 in, 2 out]
                    n153 = property on="Y" class="Slide (strict)"("Skala.Bereich:Maximum"=w410) -> ()  [unwired: 2 in, 2 out]
                    n154 = property on="Progress" class="Slide (strict)"("Scale.Maximum"=w367) -> ()  [unwired: 2 in, 2 out]
                    n155 = call "create B-Scan Stack Pattern.vi"("Size Y"="Number Scans Y", "Size X"="Number Scans X", "Range Y"=w401, "Range X"=w402, "Probe"=w400) -> ("error out"=w397:errorcluster, "Scan Pattern"=w387:refnum<class "Scan Pattern.lvclass">, "Probe"=w365:refnum<class "Probe.lvclass">)  [unwired: 2 in]
                    n156 = call "rotate Scan Pattern.vi"("error in (no error)"=w397, "Angle"="Angle [rad]", "ScanPattern"=w387) -> ("error out"=w384:errorcluster, "ScanPattern"=w390:refnum<class "Scan Pattern.lvclass">)  [unwired: 3 in]
                    n157 = property on="X" class="Slide (strict)"("Disabled"=w403) -> ()  [unwired: 2 in, 2 out]
                    n158 = property on="Y" class="Slide (strict)"("Disabled"=w403) -> ()  [unwired: 2 in, 2 out]
                    n159 = property on="Z" class="Slide (strict)"("Disabled"=w403) -> ()  [unwired: 2 in, 2 out]
                    n160 = property on="Number Scans X" class="DigNum (strict)"("Disabled"=w403) -> ()  [unwired: 2 in, 2 out]
                    n161 = property on="Number Scans Y" class="DigNum (strict)"("Disabled"=w403) -> ()  [unwired: 2 in, 2 out]
                    n162 = property on="Range X [mm]" class="DigNum (strict)"("Disabled"=w403) -> ()  [unwired: 2 in, 2 out]
                    n163 = property on="Range Y [mm]" class="DigNum (strict)"("Disabled"=w403) -> ()  [unwired: 2 in, 2 out]
                    n164 = property on="Measure" class="Bool"("Deaktiviert"=w403) -> ()  [unwired: 2 in, 2 out]
                    n165 = call "shift Scan Pattern.vi"("error in (no error)"=w384, "Shift Y"="Shift Y [mm]", "Shift X"="Shift X [mm]", "Scan Pattern in"=w390) -> ("error out"=w383:errorcluster, "Scan Pattern out"=w386:refnum<class "Scan Pattern.lvclass">)  [unwired: 2 in]
                    n166 = call "visualize Scan Pattern.vi"("error in (no error)"=w380, "Scan Pattern in"=w386, "Probe"=w365, "OCT Device"=w364) -> ("error out"=w366:errorcluster)  [unwired: 1 in, 3 out]
                    n167 = local read "Averaging Slow Axis"() -> (w370:i32)
                    n168 = call <vilib>:"Clear Errors.vi"("error in (no error)"=w366) -> ("error out"=w381:errorcluster)  [unwired: 6 in]
                    n169 = call "get Device Property Int.vi"("OCTDevice"=w392) -> ("Value"=w393:i32)  [unwired: 4 in, 2 out]
                    n170 = Merge Errors(w381, w383) -> (w382:errorcluster)
                    n171 = local read "Averaging Slow Axis"() -> (w377:i32)
                    n172 = call "create Complex Data.vi"() -> ("Complex Data"=w376:refnum<class "Complex Data.lvclass">)  [unwired: 2 in, 1 out]
                    n173 = Quotient & Remainder(x=w393, y=2) -> (floor(x/y)=w374:i32)  [unwired: 1 out]
                    n174 = call "start Measurement.vi"("error in (no error)"=w382, "Acquisition Type"=T12."Asynchronous Finite", "Scan Pattern"=w386, "OCTDevice"=w392) -> ("OCTDevice"=w385:refnum<class "OCT Device.lvclass">)  [unwired: 1 in, 2 out]
                    n175 = Multiply(x="Number Scans Y", y=w370) -> (x*y=w371:i32)
                    n176 = call "create Complex Data.vi"() -> ("Complex Data"=w379:refnum<class "Complex Data.lvclass">)  [unwired: 2 in, 1 out]
                    n177 = Tick Count (ms)() -> (millisecond timer value=w404:u32)
                    n178 = call "reserve Complex Data.vi"("Size3"=w371, "Size2"="Number Scans X", "Size1"=w374, "Complex Data in"=w376) -> ("Complex Data out"=w375:refnum<class "Complex Data.lvclass">)  [unwired: 3 in, 1 out]
                    n179 = call "create Raw Data.vi"() -> ("Raw Data"=w395:refnum<class "Raw Data.lvclass">)  [unwired: 6 in, 1 out]
                  }
                  frame #2 {
                    n180 = Multiply(x=w412, y=w426) -> (x*y=w413:i32)
                    n181 = for {
                      N: w413 -> [_]
                      tunnel: [w438] -> w425
                      tunnel: w423 -> [w447]
                      tunnel: w422 -> [w448]
                      tunnel: w421 -> [w446]
                      tunnel: w420 -> [w444]
                      tunnel: w419 -> [w431]
                      tunnel: [w430] -> w417
                      tunnel: [w440] -> w416
                      shift-right: [w442] -> w418
                      shift-left: w415 -> [w449]
                      tunnel: [w429] -> w414
                      tunnel: [w428] -> w411
                      i -> [w450]
                      n182 = call "get Raw Data.vi"("error in (no error)"=w449, "Camera Index"=0, "RawData in"=w444, "OCTDevice in"=w448) -> ("error out"=w445:errorcluster, "RawData out"=w443:refnum<class "Raw Data.lvclass">, "OCTDevice out"=w439:refnum<class "OCT Device.lvclass">)  [unwired: 1 in]
                      n183 = call-poly "set Processing Output.vi"("error in (no error)"=w445, "Complex Data in"=w447, "Processing"=w446) -> ("error out"=w441:errorcluster, "Complex Data out"=w430:refnum<class "Complex Data.lvclass">, "Processing"=w436:refnum<class "Processing.lvclass">)  [unwired: 2 in]
                      n184 = Increment(x=w450) -> (x+1=→"Progress":i32)
                      n185 = call "execute Processing.vi"("error in (no error)"=w441, "Raw Data"=w443, "Processing"=w436) -> ("error out"=w433:errorcluster, "Raw Data"=w428:refnum<class "Raw Data.lvclass">, "Processing"=w435:refnum<class "Processing.lvclass">)  [unwired: 2 in]
                      n186 = call "append Complex Data.vi"("error in (no error)"=w433, "Normal Direction"=Normal_Direction_Selection."Direction 3", "Data to append in"=w430, "Data in"=w431) -> ("error out"=w442:errorcluster, "Data to append out"=w429:refnum<class "Complex Data.lvclass">, "Data out"=w440:refnum<class "Complex Data.lvclass">)  [unwired: 1 in]
                      n187 = call "get Relative Reference Intensity.vi"("Processing"=w435, "OCTDevice"=w439) -> ("Relative Reference Intensity"=w434:dbl, "OCTDevice"=w438:refnum<class "OCT Device.lvclass">)  [unwired: 2 in, 2 out]
                      n188 = call "interpret Intensity.vi"("Intensity"=w434) -> ("Color"=w437:u32)  [unwired: 1 in, 1 out]
                      n189 = property on="Reference Intensity" class="Slide (strict)"("Fill Color"=w437) -> ()  [unwired: 2 in, 2 out]
                      n190 = local write "Reference Intensity"(w434) -> ()
                    }
                  }
                  frame #3 {
                    w475 = u8 0 ("Deaktiviert")
                    w473 = u8 0
                    n191 = local read "Averaging Fast Axis"() -> (w462:i32)
                    n192 = local read "Averaging Axially"() -> (w461:i32)
                    n193 = local read "Averaging Slow Axis"() -> (w463:i32)
                    n194 = Tick Count (ms)() -> (millisecond timer value=w476:u32)
                    n195 = call "stop Measurement.vi"("OCTDevice"=w479) -> ("OCTDevice"=w478:refnum<class "OCT Device.lvclass">)  [unwired: 5 in, 1 out]
                    n196 = call <vilib>:"Unset Busy.vi"() -> ()  [unwired: 11 in, 1 out]
                    n197 = call "clear Complex Data.vi"("Complex Data"=w465) -> ()  [unwired: 6 in, 1 out]
                    n198 = call "clear Raw Data.vi"("Raw Data"=w464) -> ()  [unwired: 6 in, 1 out]
                    n199 = call "create Speckle Variance.vi"() -> ("Speckle Variance.lvclass"=w472:refnum<class "Speckle Variance.lvclass">)  [unwired: 6 in, 1 out]
                    n200 = local read "Boundries"() -> (w456:cluster{sgl, sgl})
                    n201 = call "Benchmark.vi"("TimeStart"=w477, "NumberOfBScans"=w482, "TimeFinish"=w476) -> ("FrameRate"=→"FrameRate":sgl)  [unwired: 1 in, 2 out]
                    n202 = call <vilib>:"Simple Error Handler.vi"("error in (no error)"=w474) -> ()  [unwired: 4 in, 5 out]
                    n203 = call "set Speckle Variance Averaging.vi"("Averaging 3"=w463, "Averaging 2"=w462, "Averaging 1"=w461, "Speckle Variance in"=w472) -> ("Speckle Variance out"=w460:refnum<class "Speckle Variance.lvclass">)  [unwired: 3 in, 1 out]
                    n204 = Unbundle(w456) -> (w455:sgl, w454:sgl)
                    n205 = call "set Speckle Variance Type.vi"("Device Property Int Selection"="Variance Type", "Speckle Variance in"=w460) -> ("Speckle Variance out"=w458:refnum<class "Speckle Variance.lvclass">)  [unwired: 4 in, 1 out]
                    n206 = Max & Min(x=w455, y=w454) -> (min(x,y)=w453:sgl)  [unwired: 1 out]
                    n207 = call "set Speckle Variance Threshold.vi"("Threshold"=w453, "Speckle Variance in"=w458) -> ("Speckle Variance out"=w457:refnum<class "Speckle Variance.lvclass">)  [unwired: 4 in, 1 out]
                    n208 = call "create Data.vi"() -> ("Data"=w468:refnum<class "Data.lvclass">)  [unwired: 6 in, 1 out]
                    n209 = call "create Data.vi"() -> ("Data"=w471:refnum<class "Data.lvclass">)  [unwired: 6 in, 1 out]
                    n210 = call "compute Speckle Variance.vi"("Data Variance In"=w468, "Data Mean In"=w471, "Complex Data"=w466, "Speckle Variance in"=w457) -> ("Data Mean Out"=→"Volume Mean":refnum<class "Data.lvclass">, "Complex Data Out"=w469:refnum<class "Complex Data.lvclass">, "Data Variance Out"=→"Volume Variance":refnum<class "Data.lvclass">)  [unwired: 1 in, 2 out]
                    n211 = call "clear Complex Data.vi"("Complex Data"=w469) -> ()  [unwired: 6 in, 1 out]
                    n212 = property on="Measure" class="Bool"("Disabled"=w473) -> ()  [unwired: 2 in, 2 out]
                    n213 = property on="Recalibrate" class="Bool"("Disabled"=w473) -> ()  [unwired: 2 in, 2 out]
                    n214 = property on="Save" class="Bool"("Disabled"=w473) -> ()  [unwired: 2 in, 2 out]
                    n215 = property on="Number Scans X" class="DigNum (strict)"("Disabled"=w473) -> ()  [unwired: 2 in, 2 out]
                    n216 = property on="Number Scans Y" class="DigNum (strict)"("Disabled"=w473) -> ()  [unwired: 2 in, 2 out]
                    n217 = property on="Range X [mm]" class="DigNum (strict)"("Disabled"=w473) -> ()  [unwired: 2 in, 2 out]
                    n218 = property on="Range Y [mm]" class="DigNum (strict)"("Disabled"=w473) -> ()  [unwired: 2 in, 2 out]
                    n219 = property on="X" class="Slide (strict)"("Disabled"=w475) -> ()  [unwired: 2 in, 2 out]
                    n220 = property on="Y" class="Slide (strict)"("Disabled"=w475) -> ()  [unwired: 2 in, 2 out]
                    n221 = property on="Z" class="Slide (strict)"("Disabled"=w475) -> ()  [unwired: 2 in, 2 out]
                    n222 = property on="QuitApp" class="Bool (strict)"("Disabled"=w473) -> ()  [unwired: 2 in, 2 out]
                  }
                }
                n223 = property on="Progress" class="Slide (strict)"("Visible"=w331) -> ()  [unwired: 2 in, 2 out]
                n224 = property on="Z" class="Slide (strict)"("Val(Sgnl)"=w326) -> ()  [unwired: 2 in, 2 out]
                n225 = local write "Progress"(w332) -> ()
              }
            }
          }
          event "Test Mode": Value Change {
            n226 = event-data() -> ()  [unwired: 1 in, 1 out]
            n227 = case shown="True" "Test Mode" {
              tunnel: w488 -> [w489 w504]
              tunnel: [w489 w502] -> w486
              tunnel: w484 -> [_ w498]
              tunnel: w485 -> [_ w497]
              frame False {
              }
              frame True {
                n228 = flat-sequence {
                  tunnel: [w520] -> w507
                  tunnel: [w532] -> w505
                  tunnel: w504 -> [w531]
                  tunnel: [w528] -> w501
                  tunnel: [w524] -> w499
                  tunnel: w498 -> [w524]
                  tunnel: [w525] -> _
                  tunnel: w497 -> [w525]
                  tunnel: [w519] -> w495
                  tunnel: [w518] -> w494
                  tunnel: [w511] -> w491
                  tunnel: [w510] -> w490
                  tunnel: w505 -> [w549]
                  tunnel: [w548] -> w508
                  tunnel: w507 -> [w547]
                  tunnel: [w546] -> w506
                  tunnel: [w545] -> w503
                  tunnel: w501 -> [w544]
                  tunnel: [w544] -> w500
                  tunnel: w499 -> [w543]
                  tunnel: [w542] -> w496
                  tunnel: w495 -> [w541]
                  tunnel: w494 -> [w540]
                  tunnel: [w539] -> w493
                  tunnel: [w538] -> w492
                  tunnel: w491 -> [w537]
                  tunnel: w490 -> [w536]
                  tunnel: w508 -> [w591]
                  tunnel: w506 -> [w596]
                  tunnel: w503 -> [w594]
                  tunnel: [w595] -> w502
                  tunnel: w500 -> [w593]
                  tunnel: w496 -> [w592]
                  tunnel: w493 -> [w590]
                  tunnel: w492 -> [w589]
                  frame #0 {
                    w517 = T14."Disabled and Grayed Out" ("Disabled")
                    n229 = property on="X" class="Slide (strict)"() -> (error out=w529:errorcluster, "Disabled"=w528:u8)  [unwired: 2 in, 1 out]
                    n230 = local read "Number Scans X"() -> (w526:i32)
                    n231 = local read "Range X [mm]"() -> (w527:dbl)
                    n232 = local write "Tab Control"(enum32{"B-Scan", "Surface"}."B-Scan" ("Tab Control")) -> ()
                    n233 = property on="Averaging*Binning" class="Slide (strict)"("Disabled"=w517) -> ()  [unwired: 2 in, 2 out]
                    n234 = property on="Averaging-Binning-Ratio" class="Slide (strict)"("Disabled"=w517) -> ()  [unwired: 2 in, 2 out]
                    n235 = property on="X" class="Slide (strict)"(error in=w529, "Disabled"=w517) -> ()  [unwired: 1 in, 2 out]
                    n236 = property on="Y" class="Slide (strict)"("Disabled"=w517) -> ()  [unwired: 2 in, 2 out]
                    n237 = property on="Z" class="Slide (strict)"("Disabled"=w517) -> ()  [unwired: 2 in, 2 out]
                    n238 = property on="Measure" class="Bool"("Disabled"=w517) -> ()  [unwired: 2 in, 2 out]
                    n239 = property on="Mean Frame" class="IntGraph (strict)"("XScale.NameLbl.Text"="Width (X) [mm]" ("X Scale.Name Label.Text"), "YScale.NameLbl.Text"="Depth (Z) [mm]" ("Y Scale.Name Label.Text")) -> ()  [unwired: 2 in, 2 out]
                    n240 = call "create B-Scan Pattern.vi"("AScans"=w526, "Range"=w527, "Probe"=w525) -> ("error out"=w509:errorcluster, "Scan Pattern"=w523:refnum<class "Scan Pattern.lvclass">, "Probe"=w510:refnum<class "Probe.lvclass">)  [unwired: 3 in]
                    n241 = local read "Angle [rad]"() -> (w522:dbl)
                    n242 = local read "Shift X [mm]"() -> (w513:dbl)
                    n243 = local read "Shift Y [mm]"() -> (w512:dbl)
                    n244 = property on="Recalibrate" class="Bool"("Disabled"=w517) -> ()  [unwired: 2 in, 2 out]
                    n245 = property on="Save" class="Bool"("Disabled"=w517) -> ()  [unwired: 2 in, 2 out]
                    n246 = call "rotate Scan Pattern.vi"("error in (no error)"=w509, "Angle"=w522, "ScanPattern"=w523) -> ("error out"=w514:errorcluster, "ScanPattern"=w516:refnum<class "Scan Pattern.lvclass">)  [unwired: 3 in]
                    n247 = call "shift Scan Pattern.vi"("error in (no error)"=w514, "Shift Y"=w512, "Shift X"=w513, "Scan Pattern in"=w516) -> ("Scan Pattern out"=w515:refnum<class "Scan Pattern.lvclass">)  [unwired: 2 in, 1 out]
                    n248 = property on="Number Scans Y" class="DigNum (strict)"("Disabled"=w517) -> ()  [unwired: 2 in, 2 out]
                    n249 = property on="Range Y [mm]" class="DigNum (strict)"("Disabled"=w517) -> ()  [unwired: 2 in, 2 out]
                    n250 = property on="Range X [mm]" class="DigNum (strict)"("Disabled"=w517) -> ()  [unwired: 2 in, 2 out]
                    n251 = property on="Number Scans X" class="DigNum (strict)"("Disabled"=w517) -> ()  [unwired: 2 in, 2 out]
                    n252 = call "check for Standby.vi"("ResetTimer"=TRUE) -> ()  [unwired: 2 out]
                    n253 = call "start Measurement.vi"("error in (no error)"=w509, "Acquisition Type"=T12."Asynchronous Continuous", "Scan Pattern"=w515, "OCTDevice"=w531) -> ("error out"=w532:errorcluster, "Scan Pattern"=w511:refnum<class "Scan Pattern.lvclass">, "OCTDevice"=w520:refnum<class "OCT Device.lvclass">)  [unwired: 1 in]
                    n254 = call "create Raw Data.vi"() -> ("Raw Data"=w518:refnum<class "Raw Data.lvclass">)  [unwired: 6 in, 1 out]
                    n255 = call "create Data.vi"() -> ("Data"=w519:refnum<class "Data.lvclass">)  [unwired: 6 in, 1 out]
                  }
                  frame #1 {
                    n256 = while {
                      tunnel: w547 -> [w577]
                      tunnel: [w582] -> w546
                      tunnel: [w559] -> w545
                      tunnel: w543 -> [w575]
                      shift-right: [w558] -> w548
                      shift-left: w549 -> [w565]
                      tunnel: [w578] -> w542
                      tunnel: w541 -> [w574]
                      tunnel: w540 -> [w576]
                      tunnel: [w563] -> w539
                      tunnel: [w562] -> w538
                      tunnel: w537 -> [w555]
                      tunnel: w536 -> [w551]
                      stop <- w578 continue-if-true
                      # "Will always be \"no error\",\nbut forces order of execution."
                      n257 = call "get Raw Data.vi"("error in (no error)"=w565, "Camera Index"=0, "RawData in"=w576, "OCTDevice in"=w577) -> ("error out"=w566:errorcluster, "RawData out"=w572:refnum<class "Raw Data.lvclass">, "OCTDevice out"=w559:refnum<class "OCT Device.lvclass">)  [unwired: 1 in]
                      n258 = call-poly "set Processing Output.vi"("error in (no error)"=w565, "Data"=w574, "Processing"=w575) -> ("error out"=w571:errorcluster, "Data"=w570:refnum<class "Data.lvclass">, "Processing"=w573:refnum<class "Processing.lvclass">)  [unwired: 2 in]
                      n259 = local read "Colored Data"() -> (w560:refnum<class "Colored Data.lvclass">)
                      n260 = control-ref of="Mean Frame"() -> (w568:refnum<vi>)
                      n261 = call "execute Processing.vi"("error in (no error)"=w571, "Raw Data"=w572, "Processing"=w573) -> ("error out"=w569:errorcluster, "Raw Data"=w562:refnum<class "Raw Data.lvclass">, "Processing"=w564:refnum<class "Processing.lvclass">)  [unwired: 2 in]
                      n262 = call-poly "display Data.vi"("error in (no error)"=w569, "Data in"=w570, "IntGraph Refnum"=w568) -> ("error out"=w567:errorcluster, "Data out"=w563:refnum<class "Data.lvclass">)  [unwired: 2 in, 1 out]
                      n263 = call "get Relative Reference Intensity.vi"("Processing"=w564, "OCTDevice"=w559) -> ("Relative Reference Intensity"=w561:dbl)  [unwired: 2 in, 3 out]
                      "Reference Intensity" <- w561
                      n264 = local read "Test Mode"() -> (w586:bool)
                      n265 = local read "QuitApp"() -> (w585:bool)
                      n266 = call "interpret Intensity.vi"("Intensity"=w561) -> ("Color"=w581:u32)  [unwired: 1 in, 1 out]
                      n267 = Merge Errors(w567, w566) -> (w557:errorcluster)
                      n268 = call "get Camera Image.vi"("error in (no error)"=w557, "Colored Data in"=w560, "OCTDevice in"=w559) -> ("error out"=w554:errorcluster, "OCTDevice out"=w552:refnum<class "OCT Device.lvclass">)  [unwired: 4 in, 1 out]
                      n269 = call "visualize Scan Pattern.vi"("error in (no error)"=w554, "Scan Pattern in"=w555, "Probe"=w551, "OCT Device"=w552) -> ("error out"=w553:errorcluster)  [unwired: 1 in, 3 out]
                      n270 = call "check for Standby.vi"() -> ("TimeOut"=w582:bool)  [unwired: 1 in, 1 out]
                      n271 = Not(x=w585) -> (.not. x?=w584:bool)
                      n272 = property on="Reference Intensity" class="Slide (strict)"("Fill Color"=w581) -> ()  [unwired: 2 in, 2 out]
                      n273 = Unbundle By Name(w557) -> ("status"=w580:bool)
                      n274 = Not(x=w582) -> (.not. x?=w583:bool)
                      n275 = Not(x=w580) -> (.not. x?=w579:bool)
                      n276 = Compound Arithmetic op=AND(w586, w584, w583, w579) -> (w578:bool)
                      n277 = call <vilib>:"Clear Errors.vi"("error in (no error)"=w553) -> ("error out"=w556:errorcluster)  [unwired: 6 in]
                      n278 = Merge Errors(w557, w556) -> (w558:errorcluster)
                    }
                  }
                  frame #2 {
                    w588 = T14."Enabled" ("Disabled")
                    n279 = call "clear Data.vi"("Data"=w590) -> ()  [unwired: 6 in, 1 out]
                    n280 = call "clear Raw Data.vi"("Raw Data"=w589) -> ()  [unwired: 6 in, 1 out]
                    n281 = local write "Test Mode Indicator"(w592) -> ()
                    n282 = call <vilib>:"Simple Error Handler.vi"("error in (no error)"=w591) -> ()  [unwired: 4 in, 5 out]
                    n283 = local write "Test Mode"(w592) -> ()
                    n284 = property on="X" class="Slide (strict)"("Disabled"=w593) -> ()  [unwired: 2 in, 2 out]
                    n285 = property on="Y" class="Slide (strict)"("Disabled"=w593) -> ()  [unwired: 2 in, 2 out]
                    n286 = property on="Z" class="Slide (strict)"("Disabled"=w593) -> ()  [unwired: 2 in, 2 out]
                    n287 = property on="Measure" class="Bool"("Disabled"=w588) -> ()  [unwired: 2 in, 2 out]
                    n288 = property on="Recalibrate" class="Bool"("Disabled"=w588) -> ()  [unwired: 2 in, 2 out]
                    n289 = property on="Number Scans X" class="DigNum (strict)"("Disabled"=w588) -> ()  [unwired: 2 in, 2 out]
                    n290 = property on="Number Scans Y" class="DigNum (strict)"("Disabled"=w588) -> ()  [unwired: 2 in, 2 out]
                    n291 = property on="Range X [mm]" class="DigNum (strict)"("Disabled"=w588) -> ()  [unwired: 2 in, 2 out]
                    n292 = property on="Range Y [mm]" class="DigNum (strict)"("Disabled"=w588) -> ()  [unwired: 2 in, 2 out]
                    n293 = property on="Averaging*Binning" class="Slide (strict)"("Disabled"=w588) -> ()  [unwired: 2 in, 2 out]
                    n294 = property on="Averaging-Binning-Ratio" class="Slide (strict)"("Disabled"=w588) -> ()  [unwired: 2 in, 2 out]
                    n295 = call "activate Standby.vi"("StandBy"=w596, "OCTDevice"=w594) -> ()  [unwired: 4 in, 2 out]
                    n296 = call "stop Measurement.vi"("OCTDevice"=w594) -> ("OCTDevice"=w595:refnum<class "OCT Device.lvclass">)  [unwired: 5 in, 1 out]
                    n297 = property on="Save" class="Bool"("Disabled"=T14."Enabled") -> ()  [unwired: 2 in, 2 out]
                  }
                }
              }
            }
            "Test Mode Indicator" <- "Test Mode"
          }
          event "Tab Control": Value Change {
            n298 = event-data() -> ()  [unwired: 1 in, 6 out]
            n299 = local read "Tab Control"() -> (w597:enum32{"B-Scan"})
            n300 = case shown="\"B-Scan\", Default" w597 {
              frame "B-Scan", Default {
                w599 = u8 0 ("Deaktiviert")
                n301 = property on="X" class="Slide (strict)"("Disabled"=w599) -> ()  [unwired: 2 in, 2 out]
                n302 = property on="Y" class="Slide (strict)"("Disabled"=w599) -> ()  [unwired: 2 in, 2 out]
                n303 = property on="Z" class="Slide (strict)"("Disabled"=w599) -> ()  [unwired: 2 in, 2 out]
              }
            }
          }
          event "Range Y [mm]", "Number Scans Y", "Number Scans X", "Range X [mm]": Value Change {
            n304 = event-data() -> ()  [unwired: 1 in, 1 out]
            n305 = local read "Number Scans X"() -> (w605:i32)
            n306 = local read "Number Scans Y"() -> (w600:i32)
            n307 = Divide(x="Range X [mm]", y=w605) -> (x/y=w609:dbl)
            n308 = Divide(x="Range Y [mm]", y=w600) -> (x/y=w602:dbl)
            n309 = Multiply(x=1000.0, y=w609) -> (x*y=→"Spacing X [µm]":dbl)
            n310 = Multiply(x=1000.0, y=w602) -> (x*y=→"Spacing Y [µm]":dbl)
          }
          event "Recalibrate": Value Change {
            n311 = event-data() -> ()  [unwired: 1 in, 1 out]
            n312 = case shown="True" "Recalibrate" {
              tunnel: w612 -> [_ w616]
              tunnel: w611 -> [_ w615]
              frame False {
              }
              frame True {
                n313 = call "measure Calibration.vi"("Camera Index"=0, "Calibration Data"=Calibration_Selection."Offset Errors", "Processing"=w615, "OCTDevice"=w616) -> ()  [unwired: 2 in, 3 out]
              }
            }
          }
          event "X": Value Change {
            n314 = event-data() -> ()  [unwired: 1 in, 1 out]
            n315 = local read "Volume Variance"() -> (w635:refnum<class "Data.lvclass">)
            n316 = local read "Volume Mean"() -> (w642:refnum<class "Data.lvclass">)
            n317 = call "create Data.vi"() -> ("error out"=w633:errorcluster, "Data"=w631:refnum<class "Data.lvclass">)  [unwired: 6 in]
            n318 = call "create Data.vi"() -> ("error out"=w645:errorcluster, "Data"=w650:refnum<class "Data.lvclass">)  [unwired: 6 in]
            n319 = local read "X"() -> (w629:dbl)
            n320 = call "get Data Slice Pos.vi"("Normal Direction"=Normal_Direction_Selection."Direction 2", "error in (no error)"=w633, "Position"=w629, "Slice"=w631, "Data"=w635) -> ("error out"=w634:errorcluster, "Slice"=w637:refnum<class "Data.lvclass">)  [unwired: 2 in, 1 out]
            n321 = call "get Data Slice Pos.vi"("Normal Direction"=Normal_Direction_Selection."Direction 2", "error in (no error)"=w645, "Position"="X", "Slice"=w650, "Data"=w642) -> ("error out"=w644:errorcluster, "Slice"=w640:refnum<class "Data.lvclass">)  [unwired: 2 in, 1 out]
            n322 = local read "Filter"() -> (w636:bool)
            n323 = local read "Filter"() -> (w641:bool)
            n324 = case shown="True" w636 {
              tunnel: w637 -> [w654 w656]
              tunnel: [w654 w655] -> w638
              frame False {
              }
              frame True {
                n325 = call "Filter Bank.vi"("Data in"=w656) -> ("Data out"=w655:refnum<class "Data.lvclass">)  [unwired: 6 in]
              }
            }
            n326 = case shown="True" w641 {
              tunnel: w640 -> [w657 w659]
              tunnel: [w657 w658] -> w639
              frame False {
              }
              frame True {
                n327 = call "Filter Bank.vi"("Data in"=w659) -> ("Data out"=w658:refnum<class "Data.lvclass">)  [unwired: 6 in]
              }
            }
            n328 = control-ref of="Variance Frame"() -> (w630:refnum<vi>)
            n329 = control-ref of="Mean Frame"() -> (w647:refnum<vi>)
            n330 = call-poly "display Data.vi"("error in (no error)"=w634, "Data in"=w638, "IntGraph Refnum"=w630) -> ("error out"=w621:errorcluster, "Data out"=w622:refnum<class "Data.lvclass">)  [unwired: 2 in, 1 out]
            n331 = call-poly "display Data.vi"("error in (no error)"=w644, "Data in"=w639, "IntGraph Refnum"=w647) -> ("error out"=w643:errorcluster, "Data out"=w646:refnum<class "Data.lvclass">)  [unwired: 2 in, 1 out]
            n332 = call "clear Data.vi"("error in (no error)"=w643, "Data"=w646) -> ()  [unwired: 5 in, 1 out]
            n333 = call "analyze Data.vi"("error in (no error)"=w621, "Data Analyzation Selection"=Data_Analyzation_Selection."Min", "Data"=w622) -> ("error out"=w627:errorcluster, "Property Value"=w624:dbl, "Data out"=w625:refnum<class "Data.lvclass">)  [unwired: 2 in]
            n334 = call "analyze Data.vi"("error in (no error)"=w627, "Data Analyzation Selection"=Data_Analyzation_Selection."Max", "Data"=w625) -> ("error out"=w620:errorcluster, "Property Value"=w623:dbl, "Data out"=w619:refnum<class "Data.lvclass">)  [unwired: 2 in]
            n335 = property on="Mean Frame" class="IntGraph (strict)"("x-Achse.Namensbeschriftung.Text"="Length (Y) [mm]" ("X Scale.Name Label.Text"), "y-Achse.Namensbeschriftung.Text"="Depth (Z) [mm]" ("Y Scale.Name Label.Text")) -> ()  [unwired: 2 in, 2 out]
            n336 = property on="Variance Boundaries" class="Slide (strict)"("Scale.Minimum"=w624, "Scale.Maximum"=w623) -> (error out=w618:errorcluster)  [unwired: 2 in, 1 out]
            n337 = call <vilib>:"Clear Errors.vi"("error in (no error)"=w618) -> ()  [unwired: 6 in, 1 out]
            n338 = call "clear Data.vi"("error in (no error)"=w620, "Data"=w619) -> ()  [unwired: 5 in, 1 out]
          }
          event "Y": Value Change {
            # "Errors here might not have an influence."
            n339 = event-data() -> ()  [unwired: 1 in, 6 out]
            n340 = local read "Volume Variance"() -> (w677:refnum<class "Data.lvclass">)
            n341 = local read "Volume Mean"() -> (w684:refnum<class "Data.lvclass">)
            n342 = call "create Data.vi"() -> ("error out"=w687:errorcluster, "Data"=w694:refnum<class "Data.lvclass">)  [unwired: 6 in]
            n343 = call "create Data.vi"() -> ("error out"=w675:errorcluster, "Data"=w673:refnum<class "Data.lvclass">)  [unwired: 6 in]
            n344 = local read "Y"() -> (w672:dbl)
            n345 = call "get Data Slice Pos.vi"("Normal Direction"=Normal_Direction_Selection."Direction 3", "error in (no error)"=w687, "Position"="Y", "Slice"=w694, "Data"=w684) -> ("error out"=w686:errorcluster, "Slice"=w683:refnum<class "Data.lvclass">)  [unwired: 2 in, 1 out]
            n346 = call "get Data Slice Pos.vi"("Normal Direction"=Normal_Direction_Selection."Direction 3", "error in (no error)"=w675, "Position"=w672, "Slice"=w673, "Data"=w677) -> ("error out"=w676:errorcluster, "Slice"=w678:refnum<class "Data.lvclass">)  [unwired: 2 in, 1 out]
            n347 = local read "Filter"() -> (w681:bool)
            n348 = local read "Filter"() -> (w680:bool)
            n349 = case shown="True" w681 {
              tunnel: w683 -> [w699 w701]
              tunnel: [w699 w700] -> w682
              frame False {
              }
              frame True {
                n350 = call "Filter Bank.vi"("Data in"=w701) -> ("Data out"=w700:refnum<class "Data.lvclass">)  [unwired: 6 in]
              }
            }
            n351 = case shown="True" w680 {
              tunnel: w678 -> [w696 w698]
              tunnel: [w696 w697] -> w679
              frame False {
              }
              frame True {
                n352 = call "Filter Bank.vi"("Data in"=w698) -> ("Data out"=w697:refnum<class "Data.lvclass">)  [unwired: 6 in]
              }
            }
            n353 = control-ref of="Mean Frame"() -> (w692:refnum<vi>)
            n354 = control-ref of="Variance Frame"() -> (w671:refnum<vi>)
            n355 = call-poly "display Data.vi"("error in (no error)"=w686, "Data in"=w682, "IntGraph Refnum"=w692) -> ("error out"=w685:errorcluster, "Data out"=w691:refnum<class "Data.lvclass">)  [unwired: 2 in, 1 out]
            n356 = call-poly "display Data.vi"("error in (no error)"=w676, "Data in"=w679, "IntGraph Refnum"=w671) -> ("error out"=w661:errorcluster, "Data out"=w664:refnum<class "Data.lvclass">)  [unwired: 2 in, 1 out]
            n357 = call "clear Data.vi"("error in (no error)"=w685, "Data"=w691) -> ()  [unwired: 5 in, 1 out]
            n358 = call "analyze Data.vi"("error in (no error)"=w661, "Data Analyzation Selection"=Data_Analyzation_Selection."Min", "Data"=w664) -> ("error out"=w669:errorcluster, "Property Value"=w666:dbl, "Data out"=w667:refnum<class "Data.lvclass">)  [unwired: 2 in]
            n359 = call "analyze Data.vi"("error in (no error)"=w669, "Data Analyzation Selection"=Data_Analyzation_Selection."Max", "Data"=w667) -> ("error out"=w662:errorcluster, "Property Value"=w665:dbl, "Data out"=w663:refnum<class "Data.lvclass">)  [unwired: 2 in]
            n360 = property on="Variance Boundaries" class="Slide (strict)"("Scale.Minimum"=w666, "Scale.Maximum"=w665) -> (error out=w660:errorcluster)  [unwired: 2 in, 1 out]
            n361 = property on="Mean Frame" class="IntGraph (strict)"("x-Achse.Namensbeschriftung.Text"="Width (X) [mm]" ("X Scale.Name Label.Text"), "y-Achse.Namensbeschriftung.Text"="Depth (Z) [mm]" ("Y Scale.Name Label.Text")) -> ()  [unwired: 2 in, 2 out]
            n362 = call "clear Data.vi"("error in (no error)"=w662, "Data"=w663) -> ()  [unwired: 5 in, 1 out]
            n363 = call <vilib>:"Clear Errors.vi"("error in (no error)"=w660) -> ()  [unwired: 6 in, 1 out]
          }
          event "Z": Value Change {
            # "Errors here might not have an influence."
            n364 = event-data() -> ()  [unwired: 1 in, 1 out]
            n365 = local read "Volume Variance"() -> (w719:refnum<class "Data.lvclass">)
            n366 = local read "Volume Mean"() -> (w726:refnum<class "Data.lvclass">)
            n367 = call "create Data.vi"() -> ("error out"=w717:errorcluster, "Data"=w715:refnum<class "Data.lvclass">)  [unwired: 6 in]
            n368 = call "create Data.vi"() -> ("error out"=w729:errorcluster, "Data"=w736:refnum<class "Data.lvclass">)  [unwired: 6 in]
            n369 = local read "Z"() -> (w713:dbl)
            n370 = call "get Data Slice Pos.vi"("Normal Direction"=Normal_Direction_Selection."Direction 1", "error in (no error)"=w717, "Position"=w713, "Slice"=w715, "Data"=w719) -> ("error out"=w718:errorcluster, "Slice"=w721:refnum<class "Data.lvclass">)  [unwired: 2 in, 1 out]
            n371 = call "get Data Slice Pos.vi"("Normal Direction"=Normal_Direction_Selection."Direction 1", "error in (no error)"=w729, "Position"="Z", "Slice"=w736, "Data"=w726) -> ("error out"=w728:errorcluster, "Slice"=w724:refnum<class "Data.lvclass">)  [unwired: 2 in, 1 out]
            n372 = local read "Filter"() -> (w720:bool)
            n373 = local read "Filter"() -> (w725:bool)
            n374 = case shown="True" w720 {
              tunnel: w721 -> [w738 w740]
              tunnel: [w738 w739] -> w722
              frame False {
              }
              frame True {
                n375 = call "Filter Bank.vi"("Data in"=w740) -> ("Data out"=w739:refnum<class "Data.lvclass">)  [unwired: 6 in]
              }
            }
            n376 = case shown="True" w725 {
              tunnel: w724 -> [w741 w743]
              tunnel: [w741 w742] -> w723
              frame False {
              }
              frame True {
                n377 = call "Filter Bank.vi"("Data in"=w743) -> ("Data out"=w742:refnum<class "Data.lvclass">)  [unwired: 6 in]
              }
            }
            n378 = control-ref of="Variance Frame"() -> (w714:refnum<vi>)
            n379 = control-ref of="Mean Frame"() -> (w734:refnum<vi>)
            n380 = call-poly "display Data.vi"("error in (no error)"=w718, "Data in"=w722, "IntGraph Refnum"=w714) -> ("error out"=w711:errorcluster, "Data out"=w707:refnum<class "Data.lvclass">)  [unwired: 2 in, 1 out]
            n381 = call-poly "display Data.vi"("error in (no error)"=w728, "Data in"=w723, "IntGraph Refnum"=w734) -> ("error out"=w727:errorcluster, "Data out"=w733:refnum<class "Data.lvclass">)  [unwired: 2 in, 1 out]
            n382 = call "clear Data.vi"("error in (no error)"=w727, "Data"=w733) -> ()  [unwired: 5 in, 1 out]
            n383 = call "analyze Data.vi"("error in (no error)"=w711, "Data Analyzation Selection"=Data_Analyzation_Selection."Min", "Data"=w707) -> ("error out"=w710:errorcluster, "Property Value"=w705:dbl, "Data out"=w706:refnum<class "Data.lvclass">)  [unwired: 2 in]
            n384 = call "analyze Data.vi"("error in (no error)"=w710, "Data Analyzation Selection"=Data_Analyzation_Selection."Max", "Data"=w706) -> ("error out"=w709:errorcluster, "Property Value"=w704:dbl, "Data out"=w703:refnum<class "Data.lvclass">)  [unwired: 2 in]
            n385 = property on="Variance Boundaries" class="Slide (strict)"("Scale.Minimum"=w705, "Scale.Maximum"=w704) -> (error out=w702:errorcluster)  [unwired: 2 in, 1 out]
            n386 = property on="Mean Frame" class="IntGraph (strict)"("x-Achse.Namensbeschriftung.Text"="Width (X) [mm]" ("X Scale.Name Label.Text"), "y-Achse.Namensbeschriftung.Text"="Length (Y) [mm]" ("Y Scale.Name Label.Text")) -> ()  [unwired: 2 in, 2 out]
            n387 = call "clear Data.vi"("error in (no error)"=w709, "Data"=w703) -> ()  [unwired: 5 in, 1 out]
            n388 = call <vilib>:"Clear Errors.vi"("error in (no error)"=w702) -> ()  [unwired: 6 in, 1 out]
          }
        }
      }
      n389 = while {
        tunnel: w140 -> [w144]
        tunnel: w138 -> [w143]
        tunnel: w137 -> [w142]
        stop <- w145 stop-if-true
        n390 = event shown="[4] \"Boundries\", \"Color Scheme\": Value Change" {
          selector: _ -> [_ _ _ _ _ _ _ _ _ _ _ _]
          dyn-events: _ -> [_ _ _ _ _ _ _ _ _ _ _ _]
          timeout: 500 -> [_ _ _ _ _ _ _ _ _ _ _ _]
          tunnel: w144 -> [_ w149 _ _ _ _ w200 _ _ _ _ _]
          tunnel: w143 -> [_ w148 _ w163 _ _ _ _ _ w209 _ _]
          tunnel: w142 -> [_ w147 _ w164 _ _ _ _ _ _ _ _]
          event Timeout {
            n391 = event-data() -> ()  [unwired: 1 in, 2 out]
          }
          event "Options": Value Change {
            n392 = event-data() -> ()  [unwired: 1 in, 1 out]
            n393 = case shown="True" "Options" {
              tunnel: w148 -> [_ w156]
              tunnel: [FALSE ("Options") FALSE ("Options")] -> w151
              tunnel: w149 -> [_ w154]
              tunnel: w147 -> [_ w153]
              frame False {
              }
              frame True {
                n394 = call "Options Dialog.vi"("GalvoControl"=w153, "Processing"=w156, "OCT Device"=w154) -> ()  [unwired: 1 in]
              }
            }
            n395 = local write "Options"(w151) -> ()
          }
          event "Saturation", "Contrast", "Brightness": Value Change {
            n396 = event-data() -> ()  [unwired: 1 in, 1 out]
          }
          event "Averaging*Binning", "Averaging-Binning-Ratio", "Range X [mm]", "Number Scans X": Value Change {
            n397 = event-data() -> ()  [unwired: 1 in, 1 out]
            n398 = Decrement(x="Averaging*Binning") -> (x-1=w172:i32)
            n399 = Multiply(x=w172, y="Averaging-Binning-Ratio") -> (x*y=w169:dbl)
            n400 = To Long Integer(number=w169) -> (32bit integer=w170:i32)
            n401 = Increment(x=w172) -> (x+1=w171:i32)
            n402 = Increment(x=w170) -> (x+1=w166:i32)
            n403 = Quotient & Remainder(x=w171, y=w166) -> (floor(x/y)=w167:i32)  [unwired: 1 out]
            n404 = call "set Probe Parameter Int.vi"("Value"="Averaging*Binning", "Probe Parameter Int"=Probe_Parameter_Int_Selection."Oversampling", "GalvoControl"=w164) -> ("error out"=w159:errorcluster)  [unwired: 3 in, 1 out]
            n405 = call "set Processing Parameter Int.vi"("error in (no error)"=w159, "Value"=w167, "Processing Paramter Int Selection"=Processing_Parameter_Int_Selection."Spectrum Averaging", "Processing in"=w163) -> ("error out"=w160:errorcluster, "Processing out"=w158:refnum<class "Processing.lvclass">)  [unwired: 2 in]
            n406 = call "set Processing Parameter Int.vi"("error in (no error)"=w160, "Value"=w166, "Processing Paramter Int Selection"=Processing_Parameter_Int_Selection."A-Scan Averaging", "Processing in"=w158) -> ()  [unwired: 2 in, 2 out]
          }
          event "Boundries": Value Change {
            n407 = event-data() -> ()  [unwired: 1 in, 5 out]
            n408 = control-ref of="Mean Frame"() -> (w175:refnum<vi>)
            n409 = local read "Coloring"() -> (w182:refnum<class "Coloring.lvclass">)
            n410 = call "clear Coloring.vi"("Coloring"=w182) -> ("error out"=w179:errorcluster)  [unwired: 6 in]
            n411 = call "Palette Graph.vi"("Reference to the B-scan Graph"=w175, "Boundaries"="Boundries", "Color Scheme"="Color Scheme") -> ()
            n412 = call "create Coloring.vi"("error in (no error)"=w179, "Color Byte Order"=Coloring_Byteorder."RGBA32", "Color Table Selection"="Color Scheme") -> ("error out"=w180:errorcluster, "Coloring"=w183:refnum<class "Coloring.lvclass">)  [unwired: 3 in]
            n413 = Unbundle("Boundries") -> (w178:sgl, w177:sgl)
            n414 = call "set Coloring Boundaries.vi"("error in (no error)"=w180, "Danymic Range High [dB]"=w177, "Dynamic Range Low [dB]"=w178, "Coloring in"=w183) -> ("error out"=w174:errorcluster, "Coloring out"=w181:refnum<class "Coloring.lvclass">)  [unwired: 2 in]
            n415 = local write "Coloring"(w181) -> ()
            n416 = call <vilib>:"Simple Error Handler.vi"("error in (no error)"=w174) -> ()  [unwired: 4 in, 5 out]
          }
          event "Variance Boundaries": Value Change {
            n417 = event-data() -> ()  [unwired: 1 in, 5 out]
            n418 = control-ref of="Variance Frame"() -> (w187:refnum<vi>)
            n419 = local read "Variance Boundaries"() -> (w188:cluster{sgl, sgl})
            n420 = local read "Color Scheme"() -> (w186:T2)
            n421 = local read "Coloring"() -> (w195:refnum<class "Coloring.lvclass">)
            n422 = call "clear Coloring.vi"("Coloring"=w195) -> ("error out"=w192:errorcluster)  [unwired: 6 in]
            n423 = call "Palette Graph.vi"("Reference to the B-scan Graph"=w187, "Boundaries"=w188, "Color Scheme"=w186) -> ()
            n424 = call "create Coloring.vi"("error in (no error)"=w192, "Color Byte Order"=Coloring_Byteorder."RGBA32", "Color Table Selection"=w186) -> ("error out"=w193:errorcluster, "Coloring"=w196:refnum<class "Coloring.lvclass">)  [unwired: 3 in]
            n425 = Unbundle(w188) -> (w191:sgl, w190:sgl)
            n426 = call "set Coloring Boundaries.vi"("error in (no error)"=w193, "Danymic Range High [dB]"=w190, "Dynamic Range Low [dB]"=w191, "Coloring in"=w196) -> ("error out"=w189:errorcluster, "Coloring out"=w194:refnum<class "Coloring.lvclass">)  [unwired: 2 in]
            n427 = local write "Coloring"(w194) -> ()
            n428 = call <vilib>:"Simple Error Handler.vi"("error in (no error)"=w189) -> ()  [unwired: 4 in, 5 out]
          }
          event "Light": Value Change {
            n429 = event-data() -> ()  [unwired: 1 in, 1 out]
            n430 = call "set Output Device Value by Name.vi"("Value"="Light", "Identifier"="ring light", "OCTDevice"=w200) -> ("error out"=w197:errorcluster)  [unwired: 3 in, 1 out]
            n431 = call <vilib>:"Simple Error Handler.vi"("error in (no error)"=w197) -> ()  [unwired: 4 in, 5 out]
          }
          event Mouse Down {
            n432 = event-data() -> ()  [unwired: 1 in, 5 out]
            n433 = call "check for Standby.vi"("ResetTimer"=TRUE) -> ()  [unwired: 2 out]
          }
          event "QuitApp": Mouse Enter {
            w202 = u32 16448250
            n434 = event-data() -> ()  [unwired: 1 in, 4 out]
            n435 = Bundle(u32 16711680, u32 16448250) -> (w205:cluster{u32, u32})  [unwired: 1 in]
            n436 = Bundle(u32 8978432, w202) -> (w204:cluster{u32, u32})  [unwired: 1 in]
            n437 = Build Array(w205, w204) -> (w203:cluster{u32, u32}[])
            n438 = property on="QuitApp" class="Bool (strict)"("Colors [4]"=w203, "BoolText.TextColor"=w202) -> ()  [unwired: 2 in, 2 out]
          }
          event "Window": Value Change {
            n439 = event-data() -> ()  [unwired: 1 in, 1 out]
            n440 = call "set Apodization Window.vi"("Window"="Window", "Processing"=w209) -> ()  [unwired: 4 in, 2 out]
          }
          event "Filter Options": Value Change {
            n441 = event-data() -> ()  [unwired: 1 in, 1 out]
            n442 = case shown="True" "Filter Options" {
              frame False {
              }
              frame True {
                n443 = call "Filter Bank.vi"() -> ()  [unwired: 7 in, 1 out]
              }
            }
          }
          event "QuitApp": Mouse Leave {
            w213 = u32 0
            n444 = event-data() -> ()  [unwired: 1 in, 1 out]
            n445 = Bundle(u32 9868950, w213) -> (w214:cluster{u32, u32})  [unwired: 1 in]
            n446 = Bundle(u32 12369084, u32 0) -> (w215:cluster{u32, u32})  [unwired: 1 in]
            n447 = Build Array(w215, w214) -> (w212:cluster{u32, u32}[])
            n448 = property on="QuitApp" class="Bool (strict)"("Colors [4]"=w212, "BoolText.TextColor"=w213) -> ()  [unwired: 2 in, 2 out]
          }
        }
        n449 = local read "QuitApp"() -> (w145:bool)
      }
    }
    frame #4 {
      n450 = local read "Volume Variance"() -> (w744:refnum<class "Data.lvclass">)
      n451 = local read "Volume Mean"() -> (w745:refnum<class "Data.lvclass">)
      n452 = local read "Colored Data"() -> (w746:refnum<class "Colored Data.lvclass">)
      n453 = call "clear Data.vi"("Data"=w745) -> ()  [unwired: 6 in, 1 out]
      n454 = call "clear Data.vi"("Data"=w744) -> ()  [unwired: 6 in, 1 out]
      n455 = call "clear Colored Data.vi"("Colored Data"=w746) -> ()  [unwired: 6 in, 1 out]
    }
    frame #5 {
      n456 = call "close Device.vi"("OCTDevice"=w749) -> ()  [unwired: 6 in, 1 out]
      n457 = call "IMAQ Dispose"("All Images? (No)"=TRUE) -> ()  [unwired: 5 in, 1 out]
    }
    frame #6 {
      n458 = local read "AutoSafe"() -> (w750:bool)
      n459 = case shown="True" w750 {
        frame False {
        }
        frame True {
          n460 = local read "Number Scans X"() -> (w764:i32)
          n461 = local read "Number Scans Y"() -> (w762:i32)
          n462 = local read "Color Scheme"() -> (w751:T2)
          n463 = call "get Config Path.vi"() -> ("Path"=w752:path)  [unwired: 1 in, 1 out]
          n464 = local read "Range X [mm]"() -> (w763:dbl)
          n465 = local read "Range Y [mm]"() -> (w761:dbl)
          n466 = local read "Light"() -> (w754:i32)
          n467 = local read "Brightness"() -> (w759:sgl)
          n468 = local read "Saturation"() -> (w760:sgl)
          n469 = local read "Contrast"() -> (w758:sgl)
          n470 = local read "Window"() -> (w753:T5)
          n471 = Build Path(base path=w752, name or relative path=path "Settings.ini" ("Relative \"SpectralRadar.ini\" Path")) -> (appended path=w785:path)
          n472 = call "init Settings.vi"("Path to settings file"=w785) -> ("Settings"=w783:refnum<class "Settings.lvclass">)  [unwired: 5 in, 1 out]
          n473 = call "set Settings Entry Int.vi"("Value"=w764, "Node"="ColumnsX", "Settings"=w783) -> ("Settings"=w782:refnum<class "Settings.lvclass">)  [unwired: 3 in, 1 out]
          n474 = call "set Settings Entry Float.vi"("Value"=w763, "Node"="RangeX", "Settings"=w782) -> ("Settings"=w781:refnum<class "Settings.lvclass">)  [unwired: 3 in, 1 out]
          n475 = call "set Settings Entry Int.vi"("Value"=w762, "Node"="ColumnsY", "Settings"=w781) -> ("Settings"=w780:refnum<class "Settings.lvclass">)  [unwired: 3 in, 1 out]
          n476 = call "set Settings Entry Float.vi"("Value"=w761, "Node"="RangeY", "Settings"=w780) -> ("Settings"=w765:refnum<class "Settings.lvclass">)  [unwired: 3 in, 1 out]
          n477 = call "set Settings Entry Float.vi"("Value"=w760, "Node"="Saturation" ("Node Name"), "Settings"=w765) -> ("Settings"=w779:refnum<class "Settings.lvclass">)  [unwired: 3 in, 1 out]
          n478 = call "set Settings Entry Float.vi"("Value"=w759, "Node"="Brightness" ("Node Name"), "Settings"=w779) -> ("Settings"=w778:refnum<class "Settings.lvclass">)  [unwired: 3 in, 1 out]
          n479 = call "set Settings Entry Float.vi"("Value"=w758, "Node"="Contrast" ("Node Name"), "Settings"=w778) -> ("Settings"=w757:refnum<class "Settings.lvclass">)  [unwired: 3 in, 1 out]
          n480 = call "set Settings Entry Int.vi"("Value"=w754, "Node"="RingLight" ("Node Name"), "Settings"=w757) -> ("Settings"=w756:refnum<class "Settings.lvclass">)  [unwired: 3 in, 1 out]
          n481 = call "set Settings Entry Int.vi"("Value"=w753, "Node"="ApodizationWindow" ("Node Name"), "Settings"=w756) -> ("Settings"=w777:refnum<class "Settings.lvclass">)  [unwired: 3 in, 1 out]
          n482 = call "set Settings Entry Int.vi"("Value"=w751, "Node"="Palette" ("Node Name"), "Settings"=w777) -> ("Settings"=w776:refnum<class "Settings.lvclass">)  [unwired: 3 in, 1 out]
          n483 = call "save Settings.vi"("Settings"=w776) -> ("Settings"=w775:refnum<class "Settings.lvclass">)  [unwired: 5 in, 1 out]
          n484 = call "close Settings.vi"("Settings"=w775) -> ()  [unwired: 6 in, 1 out]
        }
      }
    }
  }
